vi "IMAQ-MWT (HOST).vi"() -> ()   [LabVIEW 2020]
uses:
  Modules/Common/Controls (HOST)/Image Size.ctl
  Modules/Common/Controls (HOST)/REF.ctl
  Modules/Common/Controls (HOST)/Image Queue Bundle.ctl
  Modules/Common/Controls (HOST)/Data to Disk Bundle.ctl
  Modules/Common/Controls (HOST)/File Name Prefix.ctl
  Modules/Common/Controls (HOST)/FPGA REF (MWT).ctl
  Modules/Common/Controls (HOST)/Experiment Mode.ctl
  Modules/Common/Controls (HOST)/Main States.ctl
  Modules/Common/Controls (HOST)/GUI Param.ctl
  Modules/Common/Controls (HOST)/Capture Background Image.ctl
  Modules/Common/Controls (HOST)/IMAQ Parameters.ctl
  Modules/Common/Controls (HOST)/File REF.ctl
  <vilib>/vision/Avi.llb/IMAQ AVI2 Refnum.ctl
  Modules/Common/Controls (HOST)/Load Parameters.ctl
  <vilib>/DAQmx/write.llb/DAQmx Write (Analog 2D DBL NChan NSamp).vi
  <vilib>/Utility/error.llb/Error Cluster From Error Code.vi
  <vilib>/rvi/errors/niLvFpgaAdjustHostInterfaceError.vi
  <vilib>/FPGAPlugInAG/Dynamic/niLvFpga_Close_Dynamic.vi
  <vilib>/Utility/file.llb/Read Delimited Spreadsheet (string).vi
  <vilib>/DAQmx/miscellaneous.llb/DAQmx Fill In Error Info.vi
  <vilib>/rvi/interface/nirviReadWriteControl/nirviReadWriteControl.xnode
  <vilib>/rvi/interface/nirviCloseFPGA/nirviCloseFPGA.xnode
  NiFpgaLv.dll
  <vilib>/rvi/interface/Simulation/niFpgaSimulationCallBeginRW.vi
  <vilib>/httpClient/LabVIEWHTTPClient.lvlib
panel:
  in  "Array Type":dbl[](array[numeric])
  in  "Record video?":bool=TRUE
  in  "File Path":path=path "D:/MWT/Data"
  in  "Display Type":enum16{"Live", "Background", "Background-Live"}(ring)
  in  "Display Frame Rate (Hz)":u32=5
  out "flipFlag":refnum<queue>
  out "Files Loaded":bool
  out "vReset":refnum<queue>
  out "FNP":T1={"DateTimeStamp"="DateTimeStamp", "Genotype 1"="genotype1", "Genotype 2"="genotype2", "Rig Name"="t21", "STIM Mode"="stimulationMode", "Light Intensity (%)"=100, "Pixel Resolution (um/pixel)"=100.0, "Gamma"=0.2, "Yoked File Name"="none", "Yoked File Enable"=FALSE, "Output Folder Name"=path "", "Frame Number"=0, "Time Stamp (us)"=0, "Exp STOP"=0, "Contour"=[], "SPINE"=[], "Larvae ID"=[], "Larvae Valid?"=[], "Image Height"=0, "Image Width"=0, "Pixel Intensity Low"=0, "Pixel Intensity High"=0, "Box Side Low"=0, "Box Side High"=0, "Box W+L Low"=0, "Box W+L High"=0, "Area Low"=0, "Area High"=0, "N SPINE"=0, "BG SUB TH"=0, "Min Contour Points"=0, "STIM Array"=[], "Stimulus Label Array"=[], "Flip Laravae ID"=[], "IR Intensity"=0}
  out "Load Options":bool
  in  "Load Settings":bool
  out "DLL Input Param":T1={"DateTimeStamp"="DateTimeStamp", "Genotype 1"="genotype1", "Genotype 2"="genotype2", "Rig Name"="t21", "STIM Mode"="stimulationMode", "Light Intensity (%)"=100, "Pixel Resolution (um/pixel)"=100.0, "Gamma"=0.2, "Yoked File Name"="none", "Yoked File Enable"=FALSE, "Output Folder Name"=path "", "Frame Number"=0, "Time Stamp (us)"=0, "Exp STOP"=0, "Contour"=[], "SPINE"=[], "Larvae ID"=[], "Larvae Valid?"=[], "Image Height"=0, "Image Width"=0, "Pixel Intensity Low"=0, "Pixel Intensity High"=0, "Box Side Low"=0, "Box Side High"=0, "Box W+L Low"=0, "Box W+L High"=0, "Area Low"=0, "Area High"=0, "N SPINE"=0, "BG SUB TH"=0, "Min Contour Points"=0, "STIM Array"=[], "Stimulus Label Array"=[], "Flip Laravae ID"=[], "IR Intensity"=0}
  in  "Tab Control":T2(tab)
  in  "Image Size":T3={"Height"=3072, "Width"=3200}
  in  "Experiment Mode":T4
  in  "Pixel Intensity Range":cluster{"Low":u8, "High":u8}={"Low"=25, "High"=135}
  in  "Exp. Time (S)":dbl=120.0
  out "Frame Rate":u32
  out "Frame #":u32
  in  "Stop Button":bool
  in  "Go":bool
  in  "Box Side (Pixels)":cluster{"Low":u32, "High":u32}={"Low"=6, "High"=200}
  out "# Objects":i32
  in  "Subtract BG":bool=TRUE
  in  "Capture BG":bool
  in  "Box W + L (Pixels)":cluster{"Low":u32, "High":u32}={"Low"=12, "High"=200}
  in  "Area (Pixels)":cluster{"Low":u32, "High":u32}={"Low"=500, "High"=3500}
  in  "Replay Interval (ms)":u32=1000
  in  "BG Type":bool=TRUE
  in  "Movie File Path":path=path "E:/Rawdata/72F11-Gal4xUAS-CsChrimson_20180513_192634.dbde"
  in  "Swap Bytes":bool
  in  "Load Stimulus":bool
  in  "STIM 10":dbl caption="unused"
  in  "STIM 9":dbl caption="unused"
  in  "STIM 8":dbl caption="unused"
  in  "STIM 7":dbl caption="unused"
  in  "STIM 6":dbl caption="unused"
  in  "STIM 5":dbl caption="unused"
  in  "STIM 4":dbl caption="testing_stim_ISI"
  in  "STIM 3":dbl caption="testing_stim_duration"
  in  "STIM 2":dbl caption="nOf_testing_stims"
  in  "STIM 1":dbl caption="Waiting_Time"
  in  "Yoke File Name":path=path "none"
  in  "Light Intensity (%)":i32=100
  in  "Yoked File Enable":bool
  in  "Save Stimulus":bool
  in  "Genotype 2":u16(ring) items=["empty-GAL4(attp2)", "UAS-CsChrimson", "LexAop-dTrpA1 VK5", " QUAS-CsCrimson(attp18)", " QUAS-dTrpA1(VK5)", " LexAop-CsChrimson (attp18)", " LexAop-CsChrimson VK5", " UAS-dTrpA1", "UAS-CsChrimsonTsh-Gal80", "UAS-CsChrimsonTH-Gal80", "UAS-CsChrimsonDdc-Gal4"]
  in  "STIM Mode":u16(ring) items=["open_loop_red", "always_on", "left_bend_continuous", "right_bend_continuous", "always_off", "random_bend_continuous_left", "random_bend_continuous_right", "bend_continuous", "forward_crawl_continuous", "open_loop_ir", "open_loop_ir_roll_dmd", "automated_assoc_learn", "two_alternatives_bend_continuous", "pulsed_ir", "DMD_IR_learning", "just_pulsed_DMD", "DMD_light_steps"]
  in  "Genotype 1":u16(ring) items=["72F11-Gal4", "72F11-LexA JK22C", " 72F11-QF2(attp2)", "11F02-Gal4", " 13xLexAop-CsChrimson_Or42b-LexA(JK22C)", " 13xLexAop-CsChrimson(attp18)_Or42b-LexA(JK22C)(ATR-)", " 13xLexAop-CsChrimson(attp18)_Or42b-LexA(JK22C)", " Or42b-LexA(JK22C)", " Or42b-Gal4", "SS04261", "58E02-Gal4", "ppk19-Gal4", "Ddc-Gal4-HL8-3D", "attP2", "w1118", "Tph-Gal4", "69F06-Gal4", "eg_gal4", "TH-Gal4", "69E06-LexALexAop-TrpA"]
  in  "Rig Name":u16(ring) items=["t21"]
  in  "Stimulus File":path=path "C:/MWT/Stimulation_Default.ini"
  in  "Settings File":path=path "C:/MWT/Settings_Default.ini"
  in  "Gamma":dbl=0.2 format="%#_13g"
  in  "Min Contour Points":u16=127
  in  "N Spine Points":fxp<+,8,8>=41.0
  in  "Pixel Resolution (um/Pixel)":dbl=40.69 format="%#_13g"
  in  "BG SUB TH":i16=50
  in  "Save Settings":bool
  in  "Cycle Time (ms)":i32=50
  in  "LASER Intensity (%)":dbl=40.0 min=0.0 max=100.0 format="%.2f"
  out "Max. LASER Power (W)":dbl format="%#.2f"
  in  "Temperature Range (High)":dbl=45.0
  in  "Temperature Range (Low)":dbl=20.0
  out "Intensity Graph":dbl[][](graph)
  out "Larvae 8":u32
  out "Larvae 7":u32
  out "Larvae 6":u32
  out "Larvae 5":u32
  out "Larvae 4":u32
  out "Larvae 3":u32
  out "Larvae 2":u32
  out "Larvae 1":u32
  out "BG Image":u8[][](array[numeric])
  out "Larvae 8":cluster{"Array":i32[], "Array":i32[]}[](graph)
  out "Larvae 7":cluster{"Array":i32[], "Array":i32[]}[](graph)
  out "Larvae 6":cluster{"Array":i32[], "Array":i32[]}[](graph)
  out "Larvae 5":cluster{"Array":i32[], "Array":i32[]}[](graph)
  out "Larvae 4":cluster{"Array":i32[], "Array":i32[]}[](graph)
  out "Larvae 3":cluster{"Array":i32[], "Array":i32[]}[](graph)
  out "Larvae 2":cluster{"Array":i32[], "Array":i32[]}[](graph)
  out "Larvae 1":cluster{"Array":i32[], "Array":i32[]}[](graph)
  out "Exp. Status":string="Camera Connected"
  out "REF":T5
  out "Command Q":refnum<queue>
  out "Display":T8(plugin-control)
  out "Stopped?":bool
  # "Real Time Multi Worm Tracker"
types:
  T1 = typedef "File Name Prefix.ctl" = cluster{"DateTimeStamp":string, "Genotype 1":string, "Genotype 2":string, "Rig Name":string, "STIM Mode":string, "Light Intensity (%)":i32, "Pixel Resolution (um/pixel)":dbl, "Gamma":dbl, "Yoked File Name":string, "Yoked File Enable":bool, "Output Folder Name":path, "Frame Number":u64, "Time Stamp (us)":u64, "Exp STOP":i32, "Contour":cluster{"X":i32[], "Y":i32[]}[], "SPINE":cluster{"X":dbl[], "Y":dbl[]}[], "Larvae ID":u32[], "Larvae Valid?":bool[], "Image Height":i32, "Image Width":i32, "Pixel Intensity Low":i32, "Pixel Intensity High":i32, "Box Side Low":i32, "Box Side High":i32, "Box W+L Low":i32, "Box W+L High":i32, "Area Low":i32, "Area High":i32, "N SPINE":i32, "BG SUB TH":i32, "Min Contour Points":i32, "STIM Array":dbl[], "Stimulus Label Array":u8[], "Flip Laravae ID":i32[], "IR Intensity":i32}
  T2 = enum32{"Experiment Setup", "Options", "Settings", "Heat Cam"}
  T3 = typedef "Image Size.ctl" = cluster{"Height":u16, "Width":u16}
  T4 = typedef "Experiment Mode.ctl" = enum16{"Live", "Replay"}
  T5 = typedef "REF.ctl" = cluster{"Queue REF":T6, "FPGA REF (MWT)":T7}
  T6 = typedef "Image Queue Bundle.ctl" = cluster{"Disk Image":refnum<queue>, "Image Blocks":refnum<queue>, "Display Image":refnum<queue>, "BG Image":refnum<queue>, "Tag Image":refnum<queue>, "DLL Input":refnum<queue>, "DMD Input":refnum<queue>, "GALVO Input":refnum<queue>, "Save Image":refnum<queue>}
  T7 = typedef "FPGA REF (MWT).ctl" = refnum<k20>
  T8 = typedef "IMAQ Image.ctl" = refnum<image>
  T9 = enum8{"Enabled", "Disabled", "Disabled and Grayed Out"}
  T10 = typedef "Main States.ctl" = enum16{"Open FPGA", "Initialize", "Preview", "Acquire Images", "STOP"}
  T11 = typedef "GUI Param.ctl" = cluster{"Image Width":u16, "Image Height":u16, "Pixel Intensity Low":u8, "Pixel Intensity High":u8, "Box Side Low":u32, "Box Side High":u32, "Box W+L Low":u32, "Box W+L High":u32, "Area Low":u32, "Area High":u32, "BG SUB TH":i16, "N Spine Points":fxp<+,8,8>, "Min Contour Points":u16, "Pixel Resolution (um/Pixel)":dbl, "Gamma":dbl}
  T12 = typedef "Load Parameters.ctl" = enum16{"Load Options", "Load Settings", "Load Stimulus", "STIM MODE"}
  T13 = typedef "IMAQ Parameters.ctl" = cluster{"File REF":T14, "Frame Data":cluster{"Width":u32, "Height":u32, "Frames Per Second":u32, "Codec":string}, "File Type":string, "Experiment Mode":T4, "Movie File Path":path}
  T14 = typedef "File REF.ctl" = cluster{"AVI REF":T15, "DBDE REF":refnum<file>}
  T15 = typedef "IMAQ AVI2 Refnum.ctl" = refnum<k20>
  T16 = typedef "Data to Disk Bundle.ctl" = cluster{"Frame Number":u64, "Time Stamp (us)":u64, "Image Data":u64[], "Contour":u32[], "Raw Image REF":refnum<data-value>, "Block Image REF":refnum<data-value>, "Block Box":u64[], "SPINE":u32[], "HT Angle":u64[], "Block Position":u64[], "SPINE Count":u32[], "Contour Count":u32[], "SPINE DIR":u8[]}
  T17 = enum16{"open", "replace", "create", "open or create", "replace or create", "replace or create with confirmation"}
  T18 = enum16{"fire", "rainbow", "gray", "inverse gray", "ice", "original"}
  T19 = typedef "Capture Background Image.ctl" = enum16{"Wait for UI", "Acquire Image", "Save Image", "Download Image"}
  T20 = enum16{"big-endian, network order", "native, host order", "little-endian"}
  T21 = typedef "IR GALVO Cal Data.ctl" = cluster{"G1X":dbl[][], "G1Y":dbl[][], "G2X":dbl[][], "G2Y":dbl[][], "G3X":dbl[][], "G3Y":dbl[][], "G4X":dbl[][], "G4Y":dbl[][], "G1 Intensity":dbl[][], "G2 Intensity":dbl[][], "G3 Intensity":dbl[][], "G4 Intensity":dbl[][], "L1 POWER":dbl[]}
  T22 = typedef "DMD Intensity Cal Param.ctl" = cluster{"X2":dbl, "X1":dbl, "C":dbl}
  T23 = typedef "imagedata.ctl" = cluster{"image type":i32, "image depth":i32, "image":u8[], "mask":u8[], "colors":u32[], "Rectangle":cluster{"left":i16, "top":i16, "right":i16, "bottom":i16}}
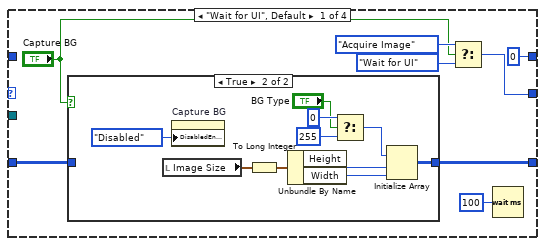
[diagram p17: hidden frame]
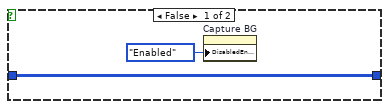
[diagram p18: hidden frame]
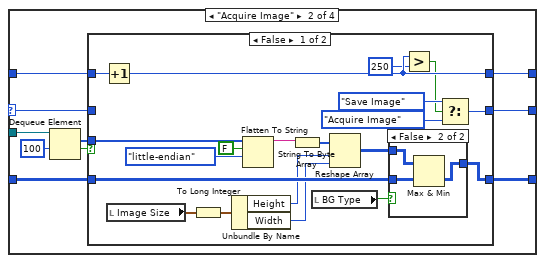
[diagram p19: hidden frame]
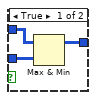
[diagram p20: hidden frame]
diagram:
  n1 = while {
    stop <- w32 stop-if-true
    # "Event Handler"
    n2 = event shown="[1] \"Go\": Value Change" {
      selector: _ -> [_ _ _ _ _ _ _ _ _ _ _]
      dyn-events: _ -> [_ _ _ _ _ _ _ _ _ _ _]
      timeout: 100 -> [_ _ _ _ _ _ _ _ _ _ _]
      event Timeout {
        n3 = event-data() -> ()  [unwired: 1 in, 1 out]
      }
      event "Go": Value Change {
        n4 = event-data() -> ("NewVal"=w33:bool)  [unwired: 1 in, 5 out]
        n5 = case shown="True" w33 {
          frame False {
          }
          frame True {
            n6 = property on="Go" class="Bool (strict)"("DisabledEnum"=T9."Disabled" ("Disabled")) -> ()  [unwired: 2 in, 2 out]
          }
        }
      }
      event "Stop Button": Value Change {
        n7 = event-data() -> ("NewVal"=w35:bool)  [unwired: 1 in]
        n8 = case shown="True" w35 {
          frame False {
          }
          frame True {
            n9 = local read "Command Q"() -> (w37:refnum<queue>)
            n10 = Enqueue Element(queue=w37, element="") -> ()  [unwired: 2 in, 3 out]
          }
        }
      }
      event "Load Options": Value Change {
        n11 = event-data() -> ()  [unwired: 1 in, 1 out]
        n12 = call "Read Options Selection (SubVI).vi"() -> ("Options Selection"=w39:i32[])  [unwired: 11 in]
        n13 = call-poly <vilib>:"Read Delimited Spreadsheet.vi"("file path (dialog if empty)"=path "C:/MWT/Options.csv", "delimiter (\\t)"="," ("delimiter (\\t)")) -> ("all rows"=w54:string[][])  [unwired: 8 in, 5 out]
        n14 = Index Array(array=w54, index (row) #1=0 ("index (row)"), index (row) #2=1 ("index (row)"), index (row) #3=2 ("index (row)"), index (row) #4=3 ("index (row)")) -> (element #1=w45:string[], element #2=w52:string[], element #3=w51:string[], element #4=w50:string[])  [unwired: 4 in]
        n15 = call "Extract Ring Text (SubVI).vi"("Spreadsheet String"=w45) -> ("Output String"=w44:string[])  [unwired: 10 in]
        n16 = call "Extract Ring Text (SubVI).vi"("Spreadsheet String"=w52) -> ("Output String"=w43:string[])  [unwired: 10 in]
        n17 = call "Extract Ring Text (SubVI).vi"("Spreadsheet String"=w51) -> ("Output String"=w42:string[])  [unwired: 10 in]
        n18 = call "Extract Ring Text (SubVI).vi"("Spreadsheet String"=w50) -> ("Output String"=w41:string[])  [unwired: 10 in]
        n19 = property on="Rig Name" class="Ring (strict)"("Strings []"=w44) -> ()  [unwired: 2 in, 2 out]
        n20 = property on="Genotype 1" class="Ring (strict)"("Strings []"=w43) -> ()  [unwired: 2 in, 2 out]
        n21 = property on="Genotype 2" class="Ring (strict)"("Strings []"=w42) -> ()  [unwired: 2 in, 2 out]
        n22 = property on="STIM Mode" class="Ring (strict)"("Strings []"=w41) -> (error out=w40:errorcluster)  [unwired: 2 in, 1 out]
        n23 = for {
          tunnel: w40 -> [_]
          tunnel: w39 -> [w56] mode=indexing
          i -> [w57]
          n24 = case shown="2" w57 {
            tunnel: w56 -> [w59 w61 w63]
            frame 0, Default {
              n25 = To Unsigned Word Integer(number=w59) -> (unsigned 16bit integer=w58:u16)
              n26 = local write "Genotype 1"(w58) -> ()
            }
            frame 1 {
              n27 = To Unsigned Word Integer(number=w61) -> (unsigned 16bit integer=w60:u16)
              n28 = local write "Genotype 2"(w60) -> ()
            }
            frame 2 {
              n29 = To Unsigned Word Integer(number=w63) -> (unsigned 16bit integer=w62:u16)
              n30 = local write "STIM Mode"(w62) -> ()
            }
          }
        }
        "Load Options" <- FALSE ("Load Options")
      }
      event "Save Settings": Value Change {
        n31 = event-data() -> ("NewVal"=w64:bool)  [unwired: 1 in]
        n32 = case shown="True" w64 {
          frame False {
          }
          frame True {
            n33 = local read "Box Side (Pixels)"() -> (w77:cluster{"Low":u32, "High":u32})
            n34 = local read "Box W + L (Pixels)"() -> (w74:cluster{"Low":u32, "High":u32})
            n35 = local read "Pixel Resolution (um/Pixel)"() -> (w68:dbl)
            n36 = local read "Image Size"() -> (w85:T3)
            n37 = local read "Pixel Intensity Range"() -> (w80:cluster{"Low":u8, "High":u8})
            n38 = local read "Area (Pixels)"() -> (w71:cluster{"Low":u32, "High":u32})
            n39 = local read "N Spine Points"() -> (w69:fxp<+,8,8>)
            n40 = local read "Min Contour Points"() -> (w67:u16)
            n41 = local read "Gamma"() -> (w66:dbl)
            n42 = local read "BG SUB TH"() -> (w70:i16)
            n43 = Unbundle By Name(w85) -> ("Width"=w84:u16, "Height"=w83:u16)
            n44 = Unbundle By Name(w80) -> ("Low"=w82:u8, "High"=w81:u8)
            n45 = Unbundle By Name(w77) -> ("Low"=w79:u32, "High"=w78:u32)
            n46 = Unbundle By Name(w74) -> ("Low"=w76:u32, "High"=w75:u32)
            n47 = Unbundle By Name(w71) -> ("Low"=w73:u32, "High"=w72:u32)
            n48 = Bundle By Name(cluster=T11 {"Image Width"=3072, "Image Height"=3072, "Pixel Intensity Low"=25, "Pixel Intensity High"=135, "Box Side Low"=6, "Box Side High"=200, "Box W+L Low"=12, "Box W+L High"=200, "Area Low"=500, "Area High"=3500, "BG SUB TH"=10, "N Spine Points"=11.0, "Min Contour Points"=127, "Pixel Resolution (um/Pixel)"=40.69, "Gamma"=0.2} ("GUI Parameters"), "Image Width"=w84, "Image Height"=w83, "Pixel Intensity Low"=w82, "Pixel Intensity High"=w81, "Box Side Low"=w79, "Box Side High"=w78, "Box W+L Low"=w76, "Box W+L High"=w75, "Area Low"=w73, "Area High"=w72, "BG SUB TH"=w70, "N Spine Points"=w69, "Min Contour Points"=w67, "Pixel Resolution (um/Pixel)"=w68, "Gamma"=w66) -> (w86:T11)
            n49 = local read "Settings File"() -> (w65:path)
            n50 = call "Save GUI Settings (SubVI).vi"("Settings File Name"=w65, "GUI Parameters"=w86) -> ()  [unwired: 10 in]
            n51 = call "Save Settings File Name (SubVI).vi"("Settings File Name"=w65) -> ()  [unwired: 11 in]
          }
        }
      }
      event "Settings File", "Load Settings": Value Change {
        n52 = event-data() -> ()  [unwired: 1 in, 6 out]
        n53 = local read "Settings File"() -> (w88:path)
        n54 = call "Read GUI Settings (SubVI).vi"("File Path"=w88) -> ("GUI Parameters"=w110:T11)  [unwired: 10 in]
        n55 = Unbundle By Name(w110) -> ("BG SUB TH"=w111:i16, "N Spine Points"=w112:fxp<+,8,8>, "Min Contour Points"=w113:u16, "Pixel Resolution (um/Pixel)"=w114:dbl, "Gamma"=w115:dbl)
        n56 = Unbundle By Name(w110) -> ("Image Width"=w92:u16, "Image Height"=w93:u16)
        n57 = Unbundle By Name(w110) -> ("Pixel Intensity Low"=w95:u8, "Pixel Intensity High"=w94:u8)
        n58 = Unbundle By Name(w110) -> ("Box Side Low"=w99:u32, "Box Side High"=w98:u32)
        n59 = Unbundle By Name(w110) -> ("Box W+L Low"=w103:u32, "Box W+L High"=w102:u32)
        n60 = Unbundle By Name(w110) -> ("Area Low"=w106:u32, "Area High"=w107:u32)
        n61 = Bundle By Name(cluster=T3 {"Height"=3072, "Width"=3072} ("Image Size"), "Width"=w92, "Height"=w93) -> (w91:T3)
        n62 = Bundle By Name(cluster=cluster{"Low":u8, "High":u8} {"Low"=25, "High"=135} ("Pixel Intensity Range"), "Low"=w95, "High"=w94) -> (w96:cluster{"Low":u8, "High":u8})
        n63 = Bundle By Name(cluster=cluster{"Low":u32, "High":u32} {"Low"=6, "High"=200} ("Box Side (Pixels)"), "Low"=w99, "High"=w98) -> (w100:cluster{"Low":u32, "High":u32})
        n64 = Bundle By Name(cluster=cluster{"Low":u32, "High":u32} {"Low"=12, "High"=200} ("Box W + L (Pixels)"), "Low"=w103, "High"=w102) -> (w105:cluster{"Low":u32, "High":u32})
        n65 = Bundle By Name(cluster=cluster{"Low":u32, "High":u32} {"Low"=500, "High"=3500} ("Area (Pixels)"), "Low"=w106, "High"=w107) -> (w109:cluster{"Low":u32, "High":u32})
        n66 = local write "Pixel Resolution (um/Pixel)"(w114) -> ()
        n67 = local write "N Spine Points"(w112) -> ()
        n68 = local write "Min Contour Points"(w113) -> ()
        n69 = local write "Gamma"(w115) -> ()
        n70 = local write "BG SUB TH"(w111) -> ()
        n71 = local write "Box Side (Pixels)"(w100) -> ()
        n72 = local write "Box W + L (Pixels)"(w105) -> ()
        n73 = local write "Image Size"(w91) -> ()
        n74 = local write "Pixel Intensity Range"(w96) -> ()
        n75 = local write "Area (Pixels)"(w109) -> ()
        n76 = local write "Load Settings"(FALSE ("Load Settings")) -> ()
      }
      event "Save Stimulus": Value Change {
        n77 = event-data() -> ("NewVal"=w116:bool)  [unwired: 1 in]
        n78 = case shown="True" w116 {
          frame False {
          }
          frame True {
            n79 = Build Array("STIM 1", "STIM 2", "STIM 3", "STIM 4", "STIM 5", "STIM 6", "STIM 7", "STIM 8", "STIM 9", "STIM 10") -> (w118:dbl[])
            n80 = property on="STIM Mode" class="Ring (strict)"() -> ("RingText.Text"=w117:string)  [unwired: 2 in, 2 out]
            n81 = local read "Stimulus File"() -> (w119:path)
            n82 = call "Save Stimulus File Name (SubVI).vi"("Stimulus File Name"=w119) -> ()  [unwired: 11 in]
            n83 = call "Save Stimulus Parameters (SubVI).vi"("STIM MODE"=w117, "Stimulus File Name"=w119, "STIM Parameters"=w118) -> ()  [unwired: 9 in]
          }
        }
      }
      event "Load Stimulus": Value Change {
        n84 = event-data() -> ("NewVal"=w130:bool)  [unwired: 1 in]
        n85 = case shown="True" w130 {
          frame False {
          }
          frame True {
            n86 = flat-sequence {
              tunnel: [w137] -> w132
              tunnel: [w133] -> w131
              tunnel: w132 -> [w165]
              tunnel: w131 -> [w163]
              frame #0 {
                n87 = local read "Stimulus File"() -> (w140:path)
                n88 = local write "Load Stimulus"(FALSE ("Load Stimulus")) -> ()
                n89 = property on="STIM Mode" class="Ring (strict)"() -> ("Strings []"=w134:string[])  [unwired: 2 in, 2 out]
                n90 = call "Load Stimulus Parameters (SubVI).vi"("Stimulus File Name"=w140) -> ("STIM MODE"=w133:string, "STIM Param"=w137:dbl[])  [unwired: 9 in]
                n91 = Search 1D Array(1D array=w134, element=w133) -> (index of element=w136:i32)  [unwired: 1 in]
                n92 = call "Read Stim Mode Labels (SubVI).vi"("STIM MODE"=w133) -> ("Label"=w138:string[])  [unwired: 10 in]
                n93 = Index Array(array=w137) -> (element #1=w150:dbl, element #2=w149:dbl, element #3=w148:dbl, element #4=w147:dbl, element #5=w146:dbl, element #6=w145:dbl, element #7=w144:dbl, element #8=w143:dbl, element #9=w142:dbl, element #10=w141:dbl)  [unwired: 10 in]
                n94 = To Unsigned Word Integer(number=w136) -> (unsigned 16bit integer=w135:u16)
                n95 = for {
                  tunnel: w138 -> [w151] mode=indexing
                  i -> [w152]
                  n96 = case shown="10" w152 {
                    tunnel: w151 -> [_ w153 w154 w155 w156 w157 w158 w159 w160 w161 w162]
                    frame 0, Default {
                    }
                    frame 1 {
                      n97 = property on="STIM 1" class="DigNum (strict)"("Caption.Text"=w153) -> ()  [unwired: 2 in, 2 out]
                    }
                    frame 2 {
                      n98 = property on="STIM 2" class="DigNum (strict)"("Caption.Text"=w154) -> ()  [unwired: 2 in, 2 out]
                    }
                    frame 3 {
                      n99 = property on="STIM 3" class="DigNum (strict)"("Caption.Text"=w155) -> ()  [unwired: 2 in, 2 out]
                    }
                    frame 4 {
                      n100 = property on="STIM 4" class="DigNum (strict)"("Caption.Text"=w156) -> ()  [unwired: 2 in, 2 out]
                    }
                    frame 5 {
                      n101 = property on="STIM 5" class="DigNum (strict)"("Caption.Text"=w157) -> ()  [unwired: 2 in, 2 out]
                    }
                    frame 6 {
                      n102 = property on="STIM 6" class="DigNum (strict)"("Caption.Text"=w158) -> ()  [unwired: 2 in, 2 out]
                    }
                    frame 7 {
                      n103 = property on="STIM 7" class="DigNum (strict)"("Caption.Text"=w159) -> ()  [unwired: 2 in, 2 out]
                    }
                    frame 8 {
                      n104 = property on="STIM 8" class="DigNum (strict)"("Caption.Text"=w160) -> ()  [unwired: 2 in, 2 out]
                    }
                    frame 9 {
                      n105 = property on="STIM 9" class="DigNum (strict)"("Caption.Text"=w161) -> ()  [unwired: 2 in, 2 out]
                    }
                    frame 10 {
                      n106 = property on="STIM 10" class="DigNum (strict)"("Caption.Text"=w162) -> ()  [unwired: 2 in, 2 out]
                    }
                  }
                }
                n107 = local write "STIM Mode"(w135) -> ()
                n108 = local write "STIM 1"(w150) -> ()
                n109 = local write "STIM 2"(w149) -> ()
                n110 = local write "STIM 3"(w148) -> ()
                n111 = local write "STIM 4"(w147) -> ()
                n112 = local write "STIM 5"(w146) -> ()
                n113 = local write "STIM 6"(w145) -> ()
                n114 = local write "STIM 7"(w144) -> ()
                n115 = local write "STIM 8"(w143) -> ()
                n116 = local write "STIM 9"(w142) -> ()
                n117 = local write "STIM 10"(w141) -> ()
              }
              frame #1 {
                n118 = for {
                  N: 10 -> [_]
                  tunnel: [w169] -> w164 mode=concatenating
                  i -> [w173]
                  n119 = case shown="0, Default" w173 {
                    tunnel: [w174 w175 w176 w177 w178 w179 w180 w181 w182 w183] -> w172
                    frame 0, Default {
                      n120 = property on="STIM 1" class="DigNum (strict)"() -> ("Caption.Text"=w174:string)  [unwired: 2 in, 2 out]
                    }
                    frame 1 {
                      n121 = property on="STIM 2" class="DigNum (strict)"() -> ("Caption.Text"=w175:string)  [unwired: 2 in, 2 out]
                    }
                    frame 2 {
                      n122 = property on="STIM 3" class="DigNum (strict)"() -> ("Caption.Text"=w176:string)  [unwired: 2 in, 2 out]
                    }
                    frame 3 {
                      n123 = property on="STIM 4" class="DigNum (strict)"() -> ("Caption.Text"=w177:string)  [unwired: 2 in, 2 out]
                    }
                    frame 4 {
                      n124 = property on="STIM 5" class="DigNum (strict)"() -> ("Caption.Text"=w178:string)  [unwired: 2 in, 2 out]
                    }
                    frame 5 {
                      n125 = property on="STIM 6" class="DigNum (strict)"() -> ("Caption.Text"=w179:string)  [unwired: 2 in, 2 out]
                    }
                    frame 6 {
                      n126 = property on="STIM 7" class="DigNum (strict)"() -> ("Caption.Text"=w180:string)  [unwired: 2 in, 2 out]
                    }
                    frame 7 {
                      n127 = property on="STIM 8" class="DigNum (strict)"() -> ("Caption.Text"=w181:string)  [unwired: 2 in, 2 out]
                    }
                    frame 8 {
                      n128 = property on="STIM 9" class="DigNum (strict)"() -> ("Caption.Text"=w182:string)  [unwired: 2 in, 2 out]
                    }
                    frame 9 {
                      n129 = property on="STIM 10" class="DigNum (strict)"() -> ("Caption.Text"=w183:string)  [unwired: 2 in, 2 out]
                    }
                  }
                  n130 = Concatenate Strings(w172, "," ("string")) -> (w171:string)
                  n131 = String To Byte Array(string=w171) -> (unsigned byte array=w169:u8[])
                }
                n132 = local read "FNP"() -> (w167:T1)
                n133 = Bundle By Name(cluster=w167, "Stimulus Label Array"=w164, "STIM Array"=w165, "STIM Mode"=w163) -> (w166:T1)
                n134 = local write "FNP"(w166) -> ()
              }
            }
          }
        }
      }
      event "Display Frame Rate (Hz)": Value Change {
        n135 = event-data() -> ()  [unwired: 1 in, 6 out]
        n136 = local read "Display Frame Rate (Hz)"() -> (w184:u32)
        n137 = call "Write Contour Display Rate (SubVI).vi"("Rate (Hz)"=w184) -> ()  [unwired: 11 in]
      }
      event "STIM Mode", "Genotype 1", "Genotype 2", "Rig Name": Value Change {
        n138 = event-data() -> ()  [unwired: 1 in, 1 out]
        n139 = flat-sequence {
          frame #0 {
            n140 = property on="STIM Mode" class="Ring (strict)"() -> ("RingText.Text"=w189:string)  [unwired: 2 in, 2 out]
            n141 = call "Read Stim Mode Labels (SubVI).vi"("STIM MODE"=w189) -> ("Label"=w190:string[])  [unwired: 10 in]
            n142 = for {
              tunnel: w190 -> [w191] mode=indexing
              i -> [w192]
              n143 = case shown="10" w192 {
                tunnel: w191 -> [_ w193 w194 w195 w196 w197 w198 w199 w200 w201 w202]
                frame 0, Default {
                }
                frame 1 {
                  n144 = property on="STIM 1" class="DigNum (strict)"("Caption.Text"=w193) -> ()  [unwired: 2 in, 2 out]
                }
                frame 2 {
                  n145 = property on="STIM 2" class="DigNum (strict)"("Caption.Text"=w194) -> ()  [unwired: 2 in, 2 out]
                }
                frame 3 {
                  n146 = property on="STIM 3" class="DigNum (strict)"("Caption.Text"=w195) -> ()  [unwired: 2 in, 2 out]
                }
                frame 4 {
                  n147 = property on="STIM 4" class="DigNum (strict)"("Caption.Text"=w196) -> ()  [unwired: 2 in, 2 out]
                }
                frame 5 {
                  n148 = property on="STIM 5" class="DigNum (strict)"("Caption.Text"=w197) -> ()  [unwired: 2 in, 2 out]
                }
                frame 6 {
                  n149 = property on="STIM 6" class="DigNum (strict)"("Caption.Text"=w198) -> ()  [unwired: 2 in, 2 out]
                }
                frame 7 {
                  n150 = property on="STIM 7" class="DigNum (strict)"("Caption.Text"=w199) -> ()  [unwired: 2 in, 2 out]
                }
                frame 8 {
                  n151 = property on="STIM 8" class="DigNum (strict)"("Caption.Text"=w200) -> ()  [unwired: 2 in, 2 out]
                }
                frame 9 {
                  n152 = property on="STIM 9" class="DigNum (strict)"("Caption.Text"=w201) -> ()  [unwired: 2 in, 2 out]
                }
                frame 10 {
                  n153 = property on="STIM 10" class="DigNum (strict)"("Caption.Text"=w202) -> ()  [unwired: 2 in, 2 out]
                }
              }
            }
          }
          frame #1 {
            n154 = property on="STIM Mode" class="Ring (strict)"() -> ("RingText.Text"=w208:string)  [unwired: 2 in, 2 out]
            n155 = property on="Genotype 1" class="Ring (strict)"() -> ("RingText.Text"=w205:string)  [unwired: 2 in, 2 out]
            n156 = property on="Genotype 2" class="Ring (strict)"() -> ("RingText.Text"=w204:string)  [unwired: 2 in, 2 out]
            n157 = property on="Rig Name" class="Ring (strict)"() -> ("RingText.Text"=w203:string)  [unwired: 2 in, 2 out]
            n158 = for {
              N: 10 -> [_]
              tunnel: [w211] -> w207 mode=concatenating
              i -> [w215]
              n159 = case shown="0, Default" w215 {
                tunnel: [w216 w217 w218 w219 w220 w221 w222 w223 w224 w225] -> w214
                frame 0, Default {
                  n160 = property on="STIM 1" class="DigNum (strict)"() -> ("Caption.Text"=w216:string)  [unwired: 2 in, 2 out]
                }
                frame 1 {
                  n161 = property on="STIM 2" class="DigNum (strict)"() -> ("Caption.Text"=w217:string)  [unwired: 2 in, 2 out]
                }
                frame 2 {
                  n162 = property on="STIM 3" class="DigNum (strict)"() -> ("Caption.Text"=w218:string)  [unwired: 2 in, 2 out]
                }
                frame 3 {
                  n163 = property on="STIM 4" class="DigNum (strict)"() -> ("Caption.Text"=w219:string)  [unwired: 2 in, 2 out]
                }
                frame 4 {
                  n164 = property on="STIM 5" class="DigNum (strict)"() -> ("Caption.Text"=w220:string)  [unwired: 2 in, 2 out]
                }
                frame 5 {
                  n165 = property on="STIM 6" class="DigNum (strict)"() -> ("Caption.Text"=w221:string)  [unwired: 2 in, 2 out]
                }
                frame 6 {
                  n166 = property on="STIM 7" class="DigNum (strict)"() -> ("Caption.Text"=w222:string)  [unwired: 2 in, 2 out]
                }
                frame 7 {
                  n167 = property on="STIM 8" class="DigNum (strict)"() -> ("Caption.Text"=w223:string)  [unwired: 2 in, 2 out]
                }
                frame 8 {
                  n168 = property on="STIM 9" class="DigNum (strict)"() -> ("Caption.Text"=w224:string)  [unwired: 2 in, 2 out]
                }
                frame 9 {
                  n169 = property on="STIM 10" class="DigNum (strict)"() -> ("Caption.Text"=w225:string)  [unwired: 2 in, 2 out]
                }
              }
              n170 = Concatenate Strings(w214, "," ("string")) -> (w213:string)
              n171 = String To Byte Array(string=w213) -> (unsigned byte array=w211:u8[])
            }
            n172 = local read "FNP"() -> (w209:T1)
            n173 = Bundle By Name(cluster=w209, "Stimulus Label Array"=w207, "STIM Mode"=w208, "Genotype 1"=w205, "Genotype 2"=w204, "Rig Name"=w203) -> (w206:T1)
            n174 = local write "FNP"(w206) -> ()
          }
        }
        n175 = Build Array("Genotype 1", "Genotype 2") -> (w186:u16[])
        n176 = To Long Integer(number=w186) -> (32bit integer=w185:i32[])
        n177 = call "Save Options Selection (SubVI).vi"("Options Selection"=w185) -> ()  [unwired: 11 in]
      }
      event "Light Intensity (%)", "Yoke File Name", "Yoked File Enable", "N Spine Points", "Min Contour Points", "Gamma", "BG SUB TH", "Pixel Resolution (um/Pixel)", "Pixel Intensity Range", "Box Side (Pixels)", "Box W + L (Pixels)", "Area (Pixels)", "STIM 1", "STIM 2", "STIM 3", "STIM 4", "STIM 5", "STIM 6", "STIM 7", "STIM 8", "STIM 9", "STIM 10": Value Change {
        n178 = event-data() -> ()  [unwired: 1 in, 6 out]
        n179 = for {
          N: 10 -> [_]
          tunnel: [w267] -> w226 mode=indexing
          i -> [w268]
          n180 = case shown="9" w268 {
            tunnel: [w269 w270 w271 w272 w273 w274 w275 w276 w277 w278] -> w267
            frame 0, Default {
              n181 = local read "STIM 1"() -> (w269:dbl)
            }
            frame 1 {
              n182 = local read "STIM 2"() -> (w270:dbl)
            }
            frame 2 {
              n183 = local read "STIM 3"() -> (w271:dbl)
            }
            frame 3 {
              n184 = local read "STIM 4"() -> (w272:dbl)
            }
            frame 4 {
              n185 = local read "STIM 5"() -> (w273:dbl)
            }
            frame 5 {
              n186 = local read "STIM 6"() -> (w274:dbl)
            }
            frame 6 {
              n187 = local read "STIM 7"() -> (w275:dbl)
            }
            frame 7 {
              n188 = local read "STIM 8"() -> (w276:dbl)
            }
            frame 8 {
              n189 = local read "STIM 9"() -> (w277:dbl)
            }
            frame 9 {
              n190 = local read "STIM 10"() -> (w278:dbl)
            }
          }
        }
        n191 = local read "Pixel Intensity Range"() -> (w237:cluster{"Low":u8, "High":u8})
        n192 = local read "Box W + L (Pixels)"() -> (w243:cluster{"Low":u32, "High":u32})
        n193 = local read "Box Side (Pixels)"() -> (w240:cluster{"Low":u32, "High":u32})
        n194 = local read "Pixel Resolution (um/Pixel)"() -> (w232:dbl)
        n195 = local read "Area (Pixels)"() -> (w246:cluster{"Low":u32, "High":u32})
        n196 = local read "Image Size"() -> (w234:T3)
        n197 = local read "Min Contour Points"() -> (w252:u16)
        n198 = local read "Light Intensity (%)"() -> (w231:i32)
        n199 = local read "Yoked File Enable"() -> (w233:bool)
        n200 = local read "Yoke File Name"() -> (w265:path)
        n201 = local read "N Spine Points"() -> (w249:fxp<+,8,8>)
        n202 = local read "BG SUB TH"() -> (w251:i16)
        n203 = local read "Gamma"() -> (w230:dbl)
        n204 = Unbundle By Name(w234) -> ("Height"=w235:u16, "Width"=w236:u16)
        n205 = Unbundle By Name(w237) -> ("Low"=w238:u8, "High"=w239:u8)
        n206 = Unbundle By Name(w240) -> ("Low"=w241:u32, "High"=w242:u32)
        n207 = Unbundle By Name(w243) -> ("Low"=w244:u32, "High"=w245:u32)
        n208 = Unbundle By Name(w246) -> ("Low"=w247:u32, "High"=w248:u32)
        n209 = To Long Integer(number=w249) -> (32bit integer=w250:i32)
        n210 = To Long Integer(number=w251) -> (32bit integer=w253:i32)
        n211 = To Long Integer(number=w252) -> (32bit integer=w254:i32)
        n212 = Path To String(path=w265) -> (string=w266:string)
        n213 = To Long Integer(number=w235) -> (32bit integer=w255:i32)
        n214 = To Long Integer(number=w236) -> (32bit integer=w256:i32)
        n215 = To Long Integer(number=w238) -> (32bit integer=w257:i32)
        n216 = To Long Integer(number=w239) -> (32bit integer=w258:i32)
        n217 = To Long Integer(number=w241) -> (32bit integer=w259:i32)
        n218 = To Long Integer(number=w242) -> (32bit integer=w260:i32)
        n219 = To Long Integer(number=w244) -> (32bit integer=w261:i32)
        n220 = To Long Integer(number=w245) -> (32bit integer=w262:i32)
        n221 = To Long Integer(number=w247) -> (32bit integer=w263:i32)
        n222 = To Long Integer(number=w248) -> (32bit integer=w264:i32)
        n223 = local read "FNP"() -> (w228:T1)
        n224 = Bundle By Name(cluster=w228, "Light Intensity (%)"=w231, "Pixel Resolution (um/pixel)"=w232, "Gamma"=w230, "Yoked File Name"=w266, "Yoked File Enable"=w233, "Image Height"=w255, "Image Width"=w256, "Pixel Intensity Low"=w257, "Pixel Intensity High"=w258, "Box Side Low"=w259, "Box Side High"=w260, "Box W+L Low"=w261, "Box W+L High"=w262, "Area Low"=w263, "Area High"=w264, "N SPINE"=w250, "BG SUB TH"=w253, "Min Contour Points"=w254, "STIM Array"=w226) -> (w229:T1)
        n225 = local write "FNP"(w229) -> ()
      }
    }
    n226 = local read "Stopped?"() -> (w32:bool)
  }
  n227 = Obtain Queue(max queue size (-1, unlimited)=10, name (unnamed)="Q", element data type="" ("name (unnamed)")) -> (queue out=→"Command Q":refnum<queue>)  [unwired: 2 in, 2 out]
  n228 = Obtain Queue(name (unnamed)="flipFlag", element data type=0) -> (queue out=→"flipFlag":refnum<queue>)  [unwired: 3 in, 2 out]
  n229 = Obtain Queue(name (unnamed)="vReset", element data type=u64 0) -> (queue out=→"vReset":refnum<queue>)  [unwired: 3 in, 2 out]
  n230 = property on="Go" class="Bool (strict)"("DisabledEnum"=T9."Enabled" ("Disabled")) -> ()  [unwired: 2 in, 2 out]
  n231 = while {
    shift-right: [w288] -> _
    shift-left: _ -> [w287]
    shift-right: [w279] -> _
    shift-left: Main_States."Open FPGA" -> [w289]
    shift-right: [w281] -> _
    shift-left: _ -> [w280]
    stop <- w285 stop-if-true
    # "Main Loop"
    n232 = case shown="\"Initialize\"" w289 {
      tunnel: [w298 w322 w343 w361 w396] -> w288
      tunnel: w287 -> [_ w323 w343 w361 w396]
      tunnel: [Main_States."Initialize" Main_States."Preview" w357 w385 Main_States."STOP"] -> w286
      tunnel: [_ _ _ _ w398] -> w285
      tunnel: [_ _ _ _ w398] -> w284
      tunnel: [w292 w327 w350 w369 w395] -> w281
      tunnel: w280 -> [_ w334 w350 w369 w395]
      frame "Open FPGA", Default {
        # "Create initial Q References"
        n233 = call "Create FPGA Reference (DBDE) (SubVI).vi"() -> ("FPGA REF (MWT)"=w300:T7)  [unwired: 11 in]
        n234 = call "Create Q Reference (SubVI).vi"() -> ("Image Queue"=w299:T6)  [unwired: 11 in]
        n235 = while {
          shift-right: [w305] -> _
          shift-left: Load_Parameters."Load Options" -> [w306]
          stop <- w304 stop-if-true
          # "Load Settings/Options/Stimulus"
          n236 = case shown="\"Load Stimulus\"" w306 {
            tunnel: [Load_Parameters."Load Settings" Load_Parameters."Load Stimulus" Load_Parameters."STIM MODE"] -> w305
            tunnel: [_ _ TRUE] -> w304
            frame "Load Options", Default {
              n237 = Wait (ms)(milliseconds to wait=u32 100) -> ()  [unwired: 1 out]
              n238 = property on="Load Options" class="Bool (strict)"("Val(Sgnl)"=TRUE ("Value (Signaling)")) -> ()  [unwired: 2 in, 2 out]
            }
            frame "Load Settings" {
              n239 = flat-sequence {
                frame #0 {
                  n240 = call "Read Settings File Name (SubVI).vi"() -> ("Settings File Name"=w312:path)  [unwired: 11 in]
                  n241 = local write "Settings File"(w312) -> ()
                }
                frame #1 {
                  n242 = property on="Load Settings" class="Bool (strict)"("Val(Sgnl)"=TRUE ("Value (Signaling)")) -> ()  [unwired: 2 in, 2 out]
                }
              }
              n243 = Wait (ms)(milliseconds to wait=u32 100) -> ()  [unwired: 1 out]
            }
            frame "Load Stimulus" {
              n244 = flat-sequence {
                frame #0 {
                  n245 = call "Read Stimulus File Name (SubVI).vi"() -> ("Stimulus File"=w317:path)  [unwired: 11 in]
                  n246 = local write "Stimulus File"(w317) -> ()
                }
                frame #1 {
                  n247 = property on="Load Stimulus" class="Bool (strict)"("Val(Sgnl)"=TRUE ("Value (Signaling)")) -> ()  [unwired: 2 in, 2 out]
                }
              }
              n248 = Wait (ms)(milliseconds to wait=u32 500) -> ()  [unwired: 1 out]
            }
          }
        }
        n249 = while {
          stop <- w303 stop-if-true
          # "Wait until DMD parameter files are loaded"
          n250 = Wait (ms)(milliseconds to wait=u32 100) -> ()  [unwired: 1 out]
          n251 = local read "Files Loaded"() -> (w303:bool)
        }
        n252 = Bundle By Name(cluster=T5 {"Queue REF"={"Disk Image"=refnum, "Image Blocks"=refnum, "Display Image"=refnum, "BG Image"=refnum, "Tag Image"=refnum, "DLL Input"=refnum, "DMD Input"=refnum, "GALVO Input"=refnum, "Save Image"=refnum}, "FPGA REF (MWT)"=refnum}, "FPGA REF (MWT)"=w300, "Queue REF"=w299) -> (w298:T5)
        "REF" <- w298
        n253 = Bundle By Name(cluster=T13 {"File REF"={"AVI REF"=refnum, "DBDE REF"=refnum}, "Frame Data"={"Width"=0, "Height"=0, "Frames Per Second"=0, "Codec"=""}, "File Type"="", "Experiment Mode"=enum."Live", "Movie File Path"=path "D:/Movies Formatted on November 5th 2015/Clip (2) Formatted.raw"} ("Movie File Property"), "Experiment Mode"="Experiment Mode", "Movie File Path"="Movie File Path") -> (w292:T13)
        n254 = local write "Exp. Status"("Please wait! Program initializing" ("Exp. Status")) -> ()
        n255 = property on="Exp. Status" class="Str"("Text.BGColor"=u32 11842560) -> ()  [unwired: 2 in, 2 out]
      }
      frame "Initialize" {
        n256 = local read "Image Size"() -> (w325:T3)
        n257 = call "Set Mode (MWT) (SubVI).vi"("Image Size In"=w325, "REF IN"=w323, "Parameters In"=w334) -> ("REF OUT"=w326:T5, "Parameters Out"=w328:T13, "Image Size Out"=w324:T3)  [unwired: 6 in]
        n258 = local write "Image Size"(w324) -> ()
        n259 = local read "Settings File"() -> (w319:path)
        n260 = call "Initialize  (MWT) (SubVI).vi"("Min Contour Points"="Min Contour Points", "N Spline Points"="N Spine Points", "REF IN"=w326, "Settings File Name"=w319, "Parameters In"=w328) -> ("REF OUT"=w322:T5, "Parameters Out"=w327:T13, "Exp. Status"=→"Exp. Status":string, "OK?"=w330:bool)  [unwired: 3 in]
        n261 = case shown="True" w330 {
          frame False {
            n262 = property on="Exp. Status" class="Str"("Text.BGColor"=u32 16729106) -> ()  [unwired: 2 in, 2 out]
          }
          frame True {
            n263 = property on="Exp. Status" class="Str"("Text.BGColor"=u32 10601373) -> ()  [unwired: 2 in, 2 out]
            n264 = local read "Command Q"() -> (w338:refnum<queue>)
            n265 = Enqueue Element(queue=w338, element="v") -> ()  [unwired: 2 in, 3 out]
          }
        }
        n266 = property on="Go" class="Bool (strict)"("DisabledEnum"=T9."Enabled" ("Disabled")) -> ()  [unwired: 2 in, 2 out]
        n267 = property on="Experiment Mode" class="Enum (strict)"("DisabledEnum"=T9."Disabled" ("Disabled")) -> ()  [unwired: 2 in, 2 out]
        n268 = local write "Go"(FALSE ("Go")) -> ()
      }
      frame "Preview" {
        # "This is where the IR camera data is gathered from the FPGA"
        n269 = local read "Experiment Mode"() -> (w341:T4)
        n270 = local read "Image Size"() -> (w347:T3)
        n271 = call "Queue Image (MMF) (SubVI).vi"("Experiment Mode"=w341, "Image Size"=w347, "Data Bundle"=w343) -> ()  [unwired: 9 in]
        n272 = Unbundle By Name(w343) -> ("FPGA REF (MWT)"=w353:T7)
        n273 = xnode "Read/Write Control"("FPGA VI Reference In"=w353, "Pixel Intensity"="Pixel Intensity Range", "Clock Cycles Limit"=u32 10000, "Swap Bytes"="Swap Bytes") -> ("Frame Interval"=w355:u32, "Frame #"=w346:u32, "DMA Timeout"=w345:bool)  [unwired: 1 in, 2 out]
        n274 = To Double Precision Float(number=w355) -> (double precision float=w354:dbl)
        n275 = local write "Frame #"(w346) -> ()
        n276 = Divide(x=110000000.0 ("y"), y=w354) -> (x/y=w351:dbl)
        n277 = To Unsigned Long Integer(number=w351) -> (unsigned 32bit integer=w349:u32)
        n278 = case shown="True" w345 {
          frame False {
          }
          frame True {
            n279 = property on="Exp. Status" class="Str"("Text.BGColor"=u32 16729106) -> ()  [unwired: 2 in, 2 out]
            n280 = local write "Exp. Status"("Reduce Frame Rate" ("Exp. Status")) -> ()
          }
        }
        n281 = local write "Frame Rate"(w349) -> ()
        n282 = Select(t=Main_States."Acquire Images", s="Go", f=Main_States."Preview") -> (s? t:f=w357:T10)
      }
      frame "Acquire Images" {
        # "Get frame index and rate"
        # "Get image data (either live or recorded)"
        # "Has total time elapsed?"
        n283 = local read "Experiment Mode"() -> (w365:T4)
        n284 = Unbundle By Name(w369) -> ("Experiment Mode"=w368:T4)
        n285 = call "Send Image to FPGA (SubVI).vi"("Data Bundle"=w361, "Parameters"=w369) -> ("TimeStamp"=w364:u64, "Frame Number"=w363:u64, "EOF"=w383:bool)  [unwired: 11 in]
        n286 = call "Queue Image (MMF) (SubVI).vi"("TimeStamp"=w364, "Frame Number"=w363, "Experiment Mode"=w365, "Image Size"="Image Size", "Data Bundle"=w361) -> ()  [unwired: 7 in]
        n287 = call "Get Elapsed Time (SubVI).vi"("Go"=TRUE, "Experiment Time (S)"="Exp. Time (S)") -> ("Done"=w374:bool, "Time Status"=w373:string)  [unwired: 8 in]
        n288 = Or(x=w374, y=w383) -> (x .or. y?=w375:bool)
        n289 = case shown="True" w383 {
          frame False {
          }
          frame True {
            n290 = One Button Dialog(message="End of Movie Reached") -> ()  [unwired: 1 in, 1 out]
          }
        }
        n291 = case shown="\"Replay\"" w368 {
          frame "Live", Default {
          }
          frame "Replay" {
            # "Limit image upload rate to 30 Hz"
            n292 = Wait (ms)(milliseconds to wait="Replay Interval (ms)") -> ()  [unwired: 1 out]
          }
        }
        n293 = local write "Exp. Status"(w373) -> ()
        n294 = local read "Pixel Intensity Range"() -> (w367:cluster{"Low":u8, "High":u8})
        n295 = Unbundle By Name(w361) -> ("FPGA REF (MWT)"=w380:T7)
        n296 = local read "Swap Bytes"() -> (w362:bool)
        n297 = xnode "Read/Write Control"("FPGA VI Reference In"=w380, "Pixel Intensity"=w367, "Significant Angle"=fxp<+,16,3> 0.0699462890625, "Swap Bytes"=w362) -> ("Frame Interval"=w382:u32, "Frame #"=→"Frame #":u32, "DMA Timeout"=w370:bool)  [unwired: 1 in, 2 out]
        n298 = case shown="True" w370 {
          frame False {
          }
          frame True {
            n299 = property on="Exp. Status" class="Str"("Text.BGColor"=u32 16729106) -> ()  [unwired: 2 in, 2 out]
            n300 = local write "Exp. Status"("Reduce Frame Rate" ("Exp. Status")) -> ()
          }
        }
        n301 = To Double Precision Float(number=w382) -> (double precision float=w381:dbl)
        n302 = Divide(x=110000000.0 ("y"), y=w381) -> (x/y=w377:dbl)
        n303 = To Unsigned Long Integer(number=w377) -> (unsigned 32bit integer=→"Frame Rate":u32)
        n304 = Select(t=Main_States."STOP", s=w375, f=Main_States."Acquire Images") -> (s? t:f=w385:T10)
      }
      frame "STOP" {
        w398 = TRUE
        n305 = Unbundle By Name(w396) -> ("FPGA REF (MWT)"=w397:T7)
        n306 = xnode "Close FPGA VI Reference"("FPGA VI Reference In"=w397) -> ("error out"=w392:errorcluster)  [unwired: 1 in]
        n307 = call <vilib>:"Clear Errors.vi"("error in (no error)"=w392) -> ()  [unwired: 5 in, 2 out]
        n308 = local write "Exp. Status"("Experiment Complete!" ("Exp. Status")) -> ()
        n309 = property on="Experiment Mode" class="Enum (strict)"("DisabledEnum"=T9."Enabled" ("Disabled")) -> ()  [unwired: 2 in, 2 out]
      }
    }
    "Stopped?" <- w284
    n310 = Select(t=Main_States."STOP", s="Stop Button", f=w286) -> (s? t:f=w279:T10)
  }
  n311 = flat-sequence {
    tunnel: [w401] -> w24
    tunnel: w24 -> [w408]
    frame #0 {
      w404 = u32 10263708 ("Plot Area:Colors:BG Color")
      # "Make sure initialization is done"
      n312 = local read "Command Q"() -> (w405:refnum<queue>)
      n313 = local write "Stopped?"(FALSE ("Stopped?")) -> ()
      n314 = local write "Files Loaded"(FALSE ("TP")) -> ()
      n315 = property on="Larvae 1" class="XYGraph (strict)"("BG Color"=w404, "FG Color"=w404, "Frame Color"=w404) -> ()  [unwired: 2 in, 2 out]
      n316 = local write "Go"(FALSE ("Go")) -> ()
      n317 = Preview Queue Element(queue=w405) -> (element=w401:string)  [unwired: 2 in, 3 out]
    }
    frame #1 {
      n318 = Equal?(x=w408, y="v") -> (x = y?=w406:bool)
      n319 = case shown="True" w406 {
        frame False {
        }
        frame True {
          w455 = 0  # Exp STOP
          # "READ EXPERIMENT DATA FROM GUI"
          n320 = for {
            N: 10 -> [_]
            tunnel: [w471] -> w415 mode=concatenating
            i -> [w475]
            n321 = case shown="0, Default" w475 {
              tunnel: [w476 w477 w478 w479 w480 w481 w482 w483 w484 w485] -> w474
              frame 0, Default {
                n322 = property on="STIM 1" class="DigNum (strict)"() -> ("Caption.Text"=w476:string)  [unwired: 2 in, 2 out]
              }
              frame 1 {
                n323 = property on="STIM 2" class="DigNum (strict)"() -> ("Caption.Text"=w477:string)  [unwired: 2 in, 2 out]
              }
              frame 2 {
                n324 = property on="STIM 3" class="DigNum (strict)"() -> ("Caption.Text"=w478:string)  [unwired: 2 in, 2 out]
              }
              frame 3 {
                n325 = property on="STIM 4" class="DigNum (strict)"() -> ("Caption.Text"=w479:string)  [unwired: 2 in, 2 out]
              }
              frame 4 {
                n326 = property on="STIM 5" class="DigNum (strict)"() -> ("Caption.Text"=w480:string)  [unwired: 2 in, 2 out]
              }
              frame 5 {
                n327 = property on="STIM 6" class="DigNum (strict)"() -> ("Caption.Text"=w481:string)  [unwired: 2 in, 2 out]
              }
              frame 6 {
                n328 = property on="STIM 7" class="DigNum (strict)"() -> ("Caption.Text"=w482:string)  [unwired: 2 in, 2 out]
              }
              frame 7 {
                n329 = property on="STIM 8" class="DigNum (strict)"() -> ("Caption.Text"=w483:string)  [unwired: 2 in, 2 out]
              }
              frame 8 {
                n330 = property on="STIM 9" class="DigNum (strict)"() -> ("Caption.Text"=w484:string)  [unwired: 2 in, 2 out]
              }
              frame 9 {
                n331 = property on="STIM 10" class="DigNum (strict)"() -> ("Caption.Text"=w485:string)  [unwired: 2 in, 2 out]
              }
            }
            n332 = Concatenate Strings(w474, "," ("string")) -> (w473:string)
            n333 = String To Byte Array(string=w473) -> (unsigned byte array=w471:u8[])
          }
          n334 = for {
            N: 10 -> [_]
            tunnel: [w486] -> w414 mode=indexing
            i -> [w487]
            n335 = case shown="9" w487 {
              tunnel: [w488 w489 w490 w491 w492 w493 w494 w495 w496 w497] -> w486
              frame 0, Default {
                n336 = local read "STIM 1"() -> (w488:dbl)
              }
              frame 1 {
                n337 = local read "STIM 2"() -> (w489:dbl)
              }
              frame 2 {
                n338 = local read "STIM 3"() -> (w490:dbl)
              }
              frame 3 {
                n339 = local read "STIM 4"() -> (w491:dbl)
              }
              frame 4 {
                n340 = local read "STIM 5"() -> (w492:dbl)
              }
              frame 5 {
                n341 = local read "STIM 6"() -> (w493:dbl)
              }
              frame 6 {
                n342 = local read "STIM 7"() -> (w494:dbl)
              }
              frame 7 {
                n343 = local read "STIM 8"() -> (w495:dbl)
              }
              frame 8 {
                n344 = local read "STIM 9"() -> (w496:dbl)
              }
              frame 9 {
                n345 = local read "STIM 10"() -> (w497:dbl)
              }
            }
          }
          n346 = local read "Movie File Path"() -> (w461:path)
          n347 = local read "Experiment Mode"() -> (w460:T4)
          n348 = local read "Pixel Intensity Range"() -> (w451:cluster{"Low":u8, "High":u8})
          n349 = local read "Box W + L (Pixels)"() -> (w445:cluster{"Low":u32, "High":u32})
          n350 = local read "Box Side (Pixels)"() -> (w448:cluster{"Low":u32, "High":u32})
          n351 = local read "Pixel Resolution (um/Pixel)"() -> (w457:dbl)
          n352 = local read "Area (Pixels)"() -> (w442:cluster{"Low":u32, "High":u32})
          n353 = local read "Image Size"() -> (w454:T3)
          n354 = local read "Min Contour Points"() -> (w436:u16)
          n355 = property on="Genotype 1" class="Ring (strict)"() -> ("RingText.Text"=w421:string)  [unwired: 2 in, 2 out]
          n356 = property on="Genotype 2" class="Ring (strict)"() -> ("RingText.Text"=w420:string)  [unwired: 2 in, 2 out]
          n357 = property on="Rig Name" class="Ring (strict)"() -> ("RingText.Text"=w419:string)  [unwired: 2 in, 2 out]
          n358 = property on="STIM Mode" class="Ring (strict)"() -> ("RingText.Text"=w418:string)  [unwired: 2 in, 2 out]
          n359 = local read "Light Intensity (%)"() -> (w458:i32)
          n360 = local read "Yoked File Enable"() -> (w456:bool)
          n361 = local read "Yoke File Name"() -> (w423:path)
          n362 = local read "N Spine Points"() -> (w439:fxp<+,8,8>)
          n363 = local read "BG SUB TH"() -> (w437:i16)
          n364 = call "Generate Date Time Stamp (SubVI).vi"("Experiment Mode"=w460, "Movie File Path"=w461) -> ("Date Time String"=w464:string)  [unwired: 9 in]
          n365 = local read "Gamma"() -> (w459:dbl)
          n366 = Unbundle By Name(w454) -> ("Height"=w453:u16, "Width"=w452:u16)
          n367 = Unbundle By Name(w451) -> ("Low"=w450:u8, "High"=w449:u8)
          n368 = Unbundle By Name(w448) -> ("Low"=w447:u32, "High"=w446:u32)
          n369 = Unbundle By Name(w445) -> ("Low"=w444:u32, "High"=w443:u32)
          n370 = Unbundle By Name(w442) -> ("Low"=w441:u32, "High"=w440:u32)
          n371 = To Long Integer(number=w439) -> (32bit integer=w438:i32)
          n372 = To Long Integer(number=w437) -> (32bit integer=w435:i32)
          n373 = To Long Integer(number=w436) -> (32bit integer=w434:i32)
          n374 = Path To String(path=w423) -> (string=w422:string)
          n375 = To Long Integer(number=w453) -> (32bit integer=w433:i32)
          n376 = To Long Integer(number=w452) -> (32bit integer=w432:i32)
          n377 = To Long Integer(number=w450) -> (32bit integer=w431:i32)
          n378 = To Long Integer(number=w449) -> (32bit integer=w430:i32)
          n379 = To Long Integer(number=w447) -> (32bit integer=w429:i32)
          n380 = To Long Integer(number=w446) -> (32bit integer=w428:i32)
          n381 = To Long Integer(number=w444) -> (32bit integer=w427:i32)
          n382 = To Long Integer(number=w443) -> (32bit integer=w426:i32)
          n383 = To Long Integer(number=w441) -> (32bit integer=w425:i32)
          n384 = To Long Integer(number=w440) -> (32bit integer=w424:i32)
          n385 = Bundle By Name(cluster=T1 {"DateTimeStamp"="DateTimeStamp", "Genotype 1"="genotype1", "Genotype 2"="genotype2", "Rig Name"="stimulationMode", "STIM Mode"="t21", "Light Intensity (%)"=100, "Pixel Resolution (um/pixel)"=100.0, "Gamma"=0.2, "Yoked File Name"="none", "Yoked File Enable"=FALSE, "Output Folder Name"=path "", "Frame Number"=0, "Time Stamp (us)"=0, "Exp STOP"=0, "Contour"=[], "SPINE"=[], "Larvae ID"=[], "Larvae Valid?"=[], "Image Height"=0, "Image Width"=0, "Pixel Intensity Low"=0, "Pixel Intensity High"=0, "Box Side Low"=0, "Box Side High"=0, "Box W+L Low"=0, "Box W+L High"=0, "Area Low"=0, "Area High"=0, "N SPINE"=0, "BG SUB TH"=0, "Min Contour Points"=0, "STIM Array"=[], "Stimulus Label Array"=[], "Flip Laravae ID"=[], "IR Intensity"=0}, "DateTimeStamp"=w464, "Genotype 1"=w421, "Genotype 2"=w420, "Rig Name"=w419, "STIM Mode"=w418, "Light Intensity (%)"=w458, "Pixel Resolution (um/pixel)"=w457, "Gamma"=w459, "Yoked File Name"=w422, "Yoked File Enable"=w456, "Exp STOP"=w455, "Image Height"=w433, "Image Width"=w432, "Pixel Intensity Low"=w431, "Pixel Intensity High"=w430, "Box Side Low"=w429, "Box Side High"=w428, "Box W+L Low"=w427, "Box W+L High"=w426, "Area Low"=w425, "Area High"=w424, "N SPINE"=w438, "BG SUB TH"=w435, "Min Contour Points"=w434, "STIM Array"=w414, "Stimulus Label Array"=w415) -> (→"FNP":T1)
          n386 = local read "REF"() -> (w409:T5)
          n387 = Unbundle By Name(w409) -> ("Queue REF.GALVO Input"=w411:refnum<queue>)
          n388 = Unbundle By Name(w409) -> ("Queue REF.Display Image"=w468:refnum<queue>)
          n389 = Unbundle By Name(w409) -> ("Queue REF.Tag Image"=w466:refnum<queue>)
          n390 = Unbundle By Name(w409) -> ("Queue REF.BG Image"=w467:refnum<queue>)
          n391 = Unbundle By Name(w409) -> ("Queue REF.Disk Image"=w469:refnum<queue>)
          n392 = Unbundle By Name(w409) -> ("Queue REF.DLL Input"=w413:refnum<queue>)
          n393 = Unbundle By Name(w409) -> ("Queue REF.DMD Input"=w412:refnum<queue>)
          n394 = Unbundle By Name(w409) -> ("Queue REF.Save Image"=w410:refnum<queue>)
          n395 = while {
            tunnel: [w511] -> w470
            tunnel: w469 -> [w503]
            tunnel: w468 -> [w510]
            tunnel: w467 -> [w508]
            tunnel: w466 -> [w507]
            tunnel: w413 -> [w502]
            tunnel: w412 -> [w501]
            tunnel: w411 -> [w500]
            tunnel: w410 -> [w499]
            stop <- w504 stop-if-true
            # "Q Images"
            n396 = property on="Stopped?" class="Bool (strict)"() -> ("Value"=w504:bool)  [unwired: 2 in, 2 out]
            n397 = Dequeue Element(queue=w503, timeout in ms (-1)=100) -> (queue out=w506:refnum<queue>, element=w509:T16, timed out?=w505:bool)  [unwired: 1 in, 1 out]
            n398 = case shown="False" w505 {
              tunnel: w506 -> [w548 w584]
              tunnel: [w548 w584] -> w511
              tunnel: w510 -> [w547 _]
              tunnel: w509 -> [w538 _]
              tunnel: w508 -> [w546 _]
              tunnel: w507 -> [w543 _]
              tunnel: w502 -> [w529 _]
              tunnel: w501 -> [w527 _]
              tunnel: w500 -> [w526 _]
              tunnel: w499 -> [w521 _]
              tunnel: "Record video?" -> [w514 _]
              frame False {
                # "Use raw image data to output contours and spines"
                # "Queue display and tag images"
                n399 = Unbundle By Name(w538) -> ("Raw Image REF"=w545:refnum<data-value>)
                n400 = Unbundle By Name(w538) -> ("Frame Number"=w518:u64, "Time Stamp (us)"=w517:u64)
                n401 = local read "LASER Intensity (%)"() -> (w525:dbl)
                n402 = for {
                  N: 128 -> [_]
                  tunnel: [w553] -> w530 mode=indexing if=w551
                  stop <- w552 stop-if-true
                  n403 = local read "flipFlag"() -> (w555:refnum<queue>)
                  n404 = Dequeue Element(queue=w555, timeout in ms (-1)=0) -> (element=w553:i32, timed out?=w552:bool)  [unwired: 1 in, 2 out]
                  n405 = Not(x=w552) -> (.not. x?=w551:bool)
                }
                n406 = local read "Capture BG"() -> (w544:bool)
                n407 = Delete Data Value Reference(data value reference=w545) -> (data value=w516:u64[])  [unwired: 1 in, 1 out]
                n408 = Bundle By Name(cluster=T16 {"Frame Number"=0, "Time Stamp (us)"=0, "Image Data"=[], "Contour"=[], "Raw Image REF"=refnum, "Block Image REF"=refnum, "Block Box"=[], "SPINE"=[], "HT Angle"=[], "Block Position"=[], "SPINE Count"=[], "Contour Count"=[], "SPINE DIR"=[]} ("element"), "Frame Number"=w518, "Time Stamp (us)"=w517, "Image Data"=w516) -> (w519:T16)
                n409 = local read "Go"() -> (w515:bool)
                n410 = Bundle By Name(cluster=w538, "Image Data"=w516) -> (w542:T16)
                n411 = call "Enque Image (BG) (SubVI).vi"("Enque"=w544, "Image Array"=w516, "BG Image REF"=w546) -> ()  [unwired: 9 in]
                n412 = local read "FNP"() -> (w532:T1)
                n413 = Bundle By Name(cluster=w532, "Frame Number"=w518, "Time Stamp (us)"=w517) -> (w539:T1)
                n414 = Multiply(x=w525, y=100.0) -> (x*y=w523:dbl)
                n415 = And(x=w514, y=w515) -> (x .and. y?=w513:bool)
                n416 = To Long Integer(number=w523) -> (32bit integer=w522:i32)
                n417 = case shown="True" w513 {
                  tunnel: w521 -> [_ w550]
                  tunnel: w519 -> [_ w549]
                  frame False {
                  }
                  frame True {
                    n418 = Enqueue Element(queue=w550, element=w549) -> ()  [unwired: 2 in, 3 out]
                  }
                }
                n419 = call "Enque Image (Display) (SubVI).vi"("Data Bundle"=w542, "Display Image REF"=w547) -> ()  [unwired: 10 in]
                n420 = call "Enque Image (Tag) (SubVI).vi"("Data Bundle"=w542, "Tag Image REF"=w543) -> ()  [unwired: 10 in]
                n421 = call "Construct Contour SPINE Array (SubVI).vi"("DATA Cluster"=w542) -> ("Larvae Valid?"=w533:bool[], "Larvae ID"=w534:u32[], "SPINE"=w535:cluster{"Array":dbl[], "Array":dbl[]}[], "Contour"=w536:cluster{"Array":i32[], "Array":i32[]}[], "Frame Valid?"=w528:bool)  [unwired: 6 in]
                n422 = Bundle By Name(cluster=w539, "Contour"=w536, "SPINE"=w535, "Larvae ID"=w534, "Larvae Valid?"=w533, "Flip Laravae ID"=w530, "IR Intensity"=w522) -> (w537:T1)
                n423 = local read "Go"() -> (w540:bool)
                n424 = And(x=w540, y=w528) -> (x .and. y?=w541:bool)
                n425 = case shown="True" w541 {
                  tunnel: w537 -> [_ w567]
                  tunnel: w529 -> [_ w564]
                  tunnel: w527 -> [_ w560]
                  tunnel: w526 -> [_ w558]
                  frame False {
                  }
                  frame True {
                    # "Update Queue REF.GALVO Input with current irData (from .dll)"
                    # "Update Queue REF.DMD Input with current dmdData (from .dll)"
                    # "Update Queue REF.DLL Input with current DLL Input Param"
                    n426 = feedback #1(TRUE ("Stopped?")) -> (w569:bool)
                    n427 = feedback-in #1(FALSE ("Stopped?")) -> ()
                    n428 = feedback #2() -> (w568:path)  [unwired: 1 in]
                    n429 = case shown="True" w569 {
                      tunnel: w567 -> [_ w582]
                      tunnel: [w580 w581] -> w566
                      tunnel: w568 -> [w580 _]
                      frame False {
                      }
                      frame True {
                        n430 = local read "Settings File"() -> (w583:path)
                        n431 = call "Create Output Folder (SubVI).vi"("Settings File Name"=w583, "DLL Input Param"=w582) -> ("Folder Name"=w581:path)  [unwired: 9 in]
                      }
                    }
                    n432 = feedback-in #2(w566) -> ()
                    n433 = Bundle By Name(cluster=w567, "Output Folder Name"=w566) -> (w563:T1)
                    "DLL Input Param" <- w563
                    n434 = Enqueue Element(queue=w564, element=w563, timeout in ms (-1)=100) -> ()  [unwired: 1 in, 3 out]
                    n435 = call "Send to Behavior Classifier (SubVI).vi"("DLL Input Param"=w563) -> ("dmdData"=w559:i32[], "voteRESET"=w565:u32[][], "irData"=w556:i32[])  [unwired: 16 in]
                    n436 = for {
                      tunnel: w565 -> [w575] mode=indexing
                      n437 = Index Array(array=w575) -> (element #1=w573:u32, element #2=w572:u32)  [unwired: 2 in]
                      n438 = Not Equal To 0?(x=w572) -> (x != 0?=w574:bool)
                      n439 = case shown="True" w574 {
                        tunnel: w573 -> [_ w578]
                        tunnel: w572 -> [_ w579]
                        frame False {
                        }
                        frame True {
                          n440 = Join Numbers(hi=w578, lo=w579) -> ((hi.lo)=w577:u64)
                          n441 = local read "vReset"() -> (w576:refnum<queue>)
                          n442 = Enqueue Element(queue=w576, element=w577) -> ()  [unwired: 2 in, 3 out]
                        }
                      }
                    }
                    n443 = Enqueue Element(queue=w560, element=w559, timeout in ms (-1)=100) -> ()  [unwired: 1 in, 3 out]
                    n444 = Enqueue Element(queue=w558, element=w556, timeout in ms (-1)=100) -> ()  [unwired: 1 in, 3 out]
                  }
                }
              }
              frame True {
              }
            }
          }
          n445 = Release Queue(queue=w470) -> (error out=w462:errorcluster)  [unwired: 2 in, 2 out]
          n446 = call <vilib>:"Clear Errors.vi"("error in (no error)"=w462) -> ()  [unwired: 5 in, 2 out]
        }
      }
    }
    frame #2 {
      n447 = local read "DLL Input Param"() -> (w587:T1)
      n448 = Bundle By Name(cluster=w587, "Exp STOP"=1) -> (w585:T1)
      n449 = local write "Stopped?"(FALSE ("Stopped?")) -> ()
      n450 = property on="Go" class="Bool (strict)"("DisabledEnum"=T9."Enabled" ("Disabled")) -> ()  [unwired: 2 in, 2 out]
      n451 = local write "Go"(FALSE ("Go")) -> ()
      n452 = call "Send to Behavior Classifier (SubVI).vi"("DLL Input Param"=w585) -> ()  [unwired: 16 in, 3 out]
    }
  }
  n453 = flat-sequence {
    tunnel: [w610] -> w17
    tunnel: [w609] -> w16
    tunnel: [w608] -> w15
    tunnel: [w595] -> w14
    tunnel: [w604] -> w13
    tunnel: [w593] -> w12
    tunnel: [w594] -> w11
    tunnel: [w603] -> w10
    tunnel: [w602] -> w9
    tunnel: [w601] -> w8
    tunnel: [w600] -> w7
    tunnel: [w599] -> w6
    tunnel: [w598] -> w5
    tunnel: [w597] -> w4
    tunnel: [w592] -> w2
    tunnel: [w591] -> w1
    tunnel: w17 -> [w664]
    tunnel: w16 -> [w663]
    tunnel: w15 -> [w662]
    tunnel: w14 -> [w661]
    tunnel: w13 -> [w660]
    tunnel: w12 -> [w658]
    tunnel: w11 -> [w659]
    tunnel: w10 -> [w657]
    tunnel: w9 -> [w656]
    tunnel: w8 -> [w651]
    tunnel: w7 -> [w650]
    tunnel: w6 -> [w645]
    tunnel: w5 -> [w644]
    tunnel: w4 -> [w643]
    tunnel: w2 -> [w641]
    tunnel: w1 -> [w634]
    frame #0 {
      # "Same as above, but for DMD 2"
      # "Initialise DMD 1 control, outputting DMD VI REF, STOP, and IMAGE REF"
      # "Wait for Qs to Initialized"
      n454 = call "Read Contour Display Rate (SubVI).vi"() -> ("Rate (Hz)"=w611:u32)  [unwired: 11 in]
      n455 = call "Read GALVO Calibration File (SubVI).vi"() -> ("GALVO Cal Data"=w591:T21)  [unwired: 11 in]
      n456 = local read "Command Q"() -> (w612:refnum<queue>)
      n457 = local write "Display Frame Rate (Hz)"(w611) -> ()
      n458 = call "Read DMD Calibration Files (SubVI).vi"() -> ("DMD2 Int"=w593:dbl[][], "DMD1 Int"=w594:dbl[][], "error out"=w596:errorcluster, "DMD1X"=w610:dbl[][], "DMD1Y"=w609:dbl[][], "DMD2X"=w608:dbl[][], "DMD2Y"=w595:dbl[][])  [unwired: 9 in]
      n459 = disable-structure shown="Disabled" {
        disable-tunnel: [w613 _] -> w597
        frame Disabled {
          n460 = Open/Create/Replace File(file path (use dialog)=path "C:/MWT/log.txt", operation (0:open)=T17."replace or create") -> (refnum out=w613:refnum<file>)  [unwired: 4 in, 2 out]
        }
        frame Enabled {
        }
      }
      n461 = call "Read DMD Calibration Parameter (SubVI).vi"() -> ("DMD Intensity Cal Param"=w592:T22)  [unwired: 11 in]
      n462 = Preview Queue Element(queue=w612) -> ()  [unwired: 2 in, 4 out]
      n463 = case shown="No Error" w596 {
        tunnel: w591 -> [_ _]
        frame No Error {
          "Files Loaded" <- TRUE ("TP")
        }
        frame Error {
        }
      }
      n464 = call "Initialize DMD 1 Control (SubVI).vi"() -> ("DMD IMG REF"=w603:refnum<vi>, "STOP REF"=w601:refnum<vi>, "DMD VI REF"=w600:refnum<vi>)  [unwired: 9 in]
      n465 = call "Initialize DMD 2 Control (SubVI).vi"() -> ("DMD IMG REF"=w602:refnum<vi>, "STOP REF"=w598:refnum<vi>, "DMD VI REF"=w599:refnum<vi>)  [unwired: 9 in]
      n466 = Initialize Array(0.0 ("element"), 768 ("dimension size"), 1024 ("dimension size")) -> (w604:dbl[][])
    }
    frame #1 {
      w624 = path "C:/Users/labadmin/Documents/projectContributors/Michael/multi-larva-cl-behavior-detection/LabViewSourceCode/heatCameraPythonCode/customFlir.py" ("module path")
      w681 = FALSE ("Save")
      # "Initialise Python session"
      # "INPUT current DMD input"
      # "From REF, insert Display Image to current code block"
      n467 = local read "REF"() -> (w665:T5)
      n468 = Unbundle By Name(w665) -> ("Queue REF.DMD Input"=w666:refnum<queue>)
      n469 = while {
        tunnel: w666 -> [w848]
        tunnel: w664 -> [w845]
        tunnel: w663 -> [w844]
        tunnel: w662 -> [w843]
        tunnel: w661 -> [w842]
        tunnel: w660 -> [w846]
        tunnel: w659 -> [w841]
        tunnel: w658 -> [w840]
        tunnel: w657 -> [w839]
        tunnel: w656 -> [w838]
        tunnel: [w837] -> w652
        tunnel: [w836] -> w649
        tunnel: w643 -> [w835]
        tunnel: [w834] -> w642
        tunnel: w641 -> [w823]
        stop <- w849 stop-if-true
        # "DMD Control Loop"
        n470 = Dequeue Element(queue=w848, timeout in ms (-1)=100) -> (element=w847:i32[], timed out?=w832:bool)  [unwired: 1 in, 2 out]
        n471 = case shown="False" w832 {
          tunnel: w847 -> [w851 _]
          tunnel: w846 -> [w869 _]
          tunnel: w845 -> [w867 _]
          tunnel: w844 -> [w866 _]
          tunnel: w843 -> [w865 _]
          tunnel: w842 -> [w864 _]
          tunnel: w841 -> [w863 _]
          tunnel: w840 -> [w862 _]
          tunnel: w839 -> [w857 _]
          tunnel: w838 -> [w856 _]
          tunnel: [w855 _] -> w837
          tunnel: [w854 _] -> w836
          tunnel: w835 -> [w853 w880]
          tunnel: [w852 w880] -> w834
          tunnel: w823 -> [w850 _]
          frame False {
            # "Get current DM stimulus parameters"
            # "Set DMD 2 REF to DMD 2 image"
            # "Set DMD 1 REF to DMD 1 image"
            n472 = local read "Pixel Resolution (um/Pixel)"() -> (w870:dbl)
            n473 = call "Rearrange DLL Output (SubVI).vi"("outData"=w851) -> ("Stimulus Parameters"=w868:dbl[][])  [unwired: 10 in]
            n474 = call "Construct DMD 1 Image (SubVI).vi"("DMD1X Array"=w867, "DMD1Y Array"=w866, "Stimulus Parameters"=w868, "DMD Intensity Cal Param"=w850, "Intensity Coefficients"=w863, "Pixel Resolution (um/Pixel)"=w870, "Initialized DMD Image Array"=w869) -> ("Image Array"=w859:u8[][])  [unwired: 12 in]
            n475 = call "Construct DMD 2 Image (SubVI).vi"("DMD2X Array"=w865, "DMD2Y Array"=w864, "Stimulus Parameters"=w868, "DMD Intensity Cal Param"=w850, "Intensity Coefficients"=w862, "Pixel Resolution (um/Pixel)"=w870, "Initialized DMD Image Array"=w869) -> ("Image Array"=w858:u8[][])  [unwired: 12 in]
            n476 = disable-structure shown="Disabled" {
              disable-tunnel: w853 -> [w876 _]
              disable-tunnel: [w874 _] -> w852
              frame Disabled {
                n477 = Get Date/Time In Seconds() -> (seconds since 1Jan1904=w875:timestamp)
                n478 = To Double Precision Float(number=w875) -> (double precision float=w871:dbl)
                n479 = feedback #3(w871) -> (w872:dbl)
                n480 = feedback-in #3(w871) -> ()
                n481 = Subtract(x=w871, y=w872) -> (x-y=w873:dbl)
                n482 = Number To Fractional String(number=w873) -> (F-format string=w877:string)  [unwired: 3 in]
                n483 = Concatenate Strings(w877, "\r\n") -> (w878:string)
                n484 = Write to Text File(file (use dialog)=w876, text=w878) -> (refnum out=w874:refnum<file>)  [unwired: 2 in, 2 out]
              }
              frame Enabled {
              }
            }
            n485 = To Variant(anything=w859) -> (Variant=w861:variant)
            n486 = To Variant(anything=w858) -> (Variant=w860:variant)
            n487 = property class="Ctl"(reference=w857, "Value"=w861) -> (error out=w855:errorcluster)  [unwired: 1 in, 1 out]
            n488 = property class="Ctl"(reference=w856, "Value"=w860) -> (error out=w854:errorcluster)  [unwired: 1 in, 1 out]
          }
          frame True {
          }
        }
        n489 = local read "Frame Rate"() -> (w825:u32)
        n490 = Greater Than 0?(x=w825) -> (x > 0?=w826:bool)
        n491 = Select(t=w825, s=w826, f=u32 1) -> (s? t:f=w827:u32)
        n492 = To Double Precision Float(number=w827) -> (double precision float=w831:dbl)
        n493 = Divide(x=1000.0, y=w831) -> (x/y=w829:dbl)
        n494 = To Unsigned Long Integer(number=w829) -> (unsigned 32bit integer=w828:u32)
        n495 = Wait Until Next ms Multiple(millisecond multiple=w828) -> ()  [unwired: 1 out]
        n496 = property on="Stopped?" class="Bool (strict)"() -> ("Value"=w849:bool)  [unwired: 2 in, 2 out]
      }
      n497 = disable-structure shown="Disabled" {
        disable-tunnel: w642 -> [w822 _]
        frame Disabled {
          n498 = Close File(refnum=w822) -> ()  [unwired: 1 in, 2 out]
        }
        frame Enabled {
        }
      }
      n499 = To Variant(anything=TRUE ("Wait Until Done")) -> (Variant=w654:variant)
      n500 = To Variant(anything=TRUE ("Wait Until Done")) -> (Variant=w647:variant)
      n501 = property class="Ctl"(reference=w651, error in=w652, "Value"=w654) -> (error out=w653:errorcluster)  [unwired: 1 out]
      n502 = property class="Ctl"(reference=w644, error in=w649, "Value"=w647) -> (error out=w648:errorcluster)  [unwired: 1 out]
      n503 = invoke class="VI" method="FP.Close"(reference=w650, error in=w653) -> ()  [unwired: 1 in, 3 out]
      n504 = invoke class="VI" method="FP.Close"(reference=w645, error in=w648) -> ()  [unwired: 1 in, 3 out]
      n505 = local read "REF"() -> (w668:T5)
      n506 = Unbundle By Name(w668) -> ("Queue REF.Display Image"=w669:refnum<queue>)
      n507 = call "Create AVI FName (SubVI).vi"("Save"=w681) -> ("Image REF"=w678:T8, "AVI Refnum"=w679:T15)  [unwired: 9 in]
      n508 = while {
        tunnel: [w1013] -> w667
        tunnel: w669 -> [w1012]
        tunnel: w679 -> [w1009]
        tunnel: [w1008] -> w671
        tunnel: w678 -> [w1007]
        tunnel: w681 -> [w1006]
        tunnel: w681 -> [w1005]
        stop <- w1010 stop-if-true
        # "Take an image and pass it on every 100 ms?"
        # "Case structure: is testing on?"
        # "Display Image"
        n509 = property on="Stopped?" class="Bool (strict)"() -> ("Value"=w1010:bool)  [unwired: 2 in, 2 out]
        n510 = Dequeue Element(queue=w1012, timeout in ms (-1)=100) -> (queue out=w1014:refnum<queue>, element=w1011:T16, timed out?=w1015:bool)  [unwired: 1 in, 1 out]
        n511 = case shown="False" w1015 {
          tunnel: w1014 -> [w1024 w1097]
          tunnel: [w1024 w1097] -> w1013
          tunnel: w1011 -> [w1023 _]
          tunnel: w1009 -> [w1022 w1096]
          tunnel: [w1021 w1096] -> w1008
          tunnel: w1007 -> [w1020 _]
          tunnel: w1006 -> [w1018 _]
          tunnel: w1005 -> [w1017 _]
          frame False {
            # "MAIN PROGRAM CODE"
            # "Testing code to save progam GUI screeshots to .avi"
            n512 = flat-sequence {
              tunnel: w1023 -> [w1031]
              tunnel: [w1091] -> w1019
              tunnel: w1017 -> [w1090]
              frame #0 {
                # "Only if > 0"
                # "Set (slow) frame rate for displaying larva outlines (default = 5 Hz)"
                # "DISPLAY DETECTED LARVA OUTLINES / SPINES"
                # "Display image"
                # "SHOW LIVE / BG / BG-SUBTRACTED IMAGE\nCase structure which determines what image will be displayed, based on input from Display Type"
                # "GUI button to select display type"
                n513 = Greater Than 0?(x="Display Frame Rate (Hz)") -> (x > 0?=w1034:bool)
                n514 = case shown="True" w1034 {
                  tunnel: w1031 -> [_ w1066]
                  tunnel: "Display Frame Rate (Hz)" -> [_ w1056]
                  frame False {
                  }
                  frame True {
                    # "Take display data and return contour, spine, head, tail, and ID data"
                    # "For loop to display larva outlines (1-8)"
                    # "Calculate ms to wait (from Hz)"
                    # "Convert to double precision"
                    n515 = call "Display Contour SPINE Head Tail (SubVI).vi"("Display Data"=w1066) -> ("Contour Array"=w1065:cluster{"Array":i32[], "Array":i32[]}[], "SPINE Array"=w1064:cluster{"Array":i32[], "Array":i32[]}[], "Head Array"=w1063:cluster{"Array":i32[], "Array":i32[]}[], "Tail Array"=w1062:cluster{"Array":i32[], "Array":i32[]}[], "Larvae ID"=w1061:u32[])  [unwired: 10 in]
                    n516 = for {
                      tunnel: w1065 -> [w1073] mode=indexing
                      tunnel: w1064 -> [w1072] mode=indexing
                      tunnel: w1063 -> [w1071] mode=indexing
                      tunnel: w1062 -> [w1070] mode=indexing
                      tunnel: w1061 -> [w1067] mode=indexing
                      i -> [w1068]
                      # "i = iteration count"
                      # "Combine outlines/spines/etc data into single array"
                      n517 = Build Array(w1073, w1072, w1071, w1070) -> (w1069:cluster{"Array":i32[], "Array":i32[]}[])
                      n518 = case shown="2" w1068 {
                        tunnel: w1069 -> [w1075 w1077 w1079 w1081 w1083 w1085 w1087 w1089 _]
                        tunnel: w1067 -> [w1074 w1076 w1078 w1080 w1082 w1084 w1086 w1088 _]
                        frame 0 {
                          # "Show outlines"
                          # "Show larva ID"
                          "Larvae 1" <- w1075
                          "Larvae 1" <- w1074
                        }
                        frame 1 {
                          "Larvae 2" <- w1077
                          "Larvae 2" <- w1076
                        }
                        frame 2 {
                          "Larvae 3" <- w1079
                          "Larvae 3" <- w1078
                        }
                        frame 3 {
                          "Larvae 4" <- w1081
                          "Larvae 4" <- w1080
                        }
                        frame 4 {
                          "Larvae 5" <- w1083
                          "Larvae 5" <- w1082
                        }
                        frame 5 {
                          "Larvae 6" <- w1085
                          "Larvae 6" <- w1084
                        }
                        frame 6 {
                          "Larvae 7" <- w1087
                          "Larvae 7" <- w1086
                        }
                        frame 7 {
                          "Larvae 8" <- w1089
                          "Larvae 8" <- w1088
                        }
                        frame 8, Default {
                        }
                      }
                    }
                    n519 = To Double Precision Float(number=w1056) -> (double precision float=w1057:dbl)
                    n520 = Divide(x=1000.0, y=w1057) -> (x/y=w1058:dbl)
                    n521 = To Unsigned Long Integer(number=w1058) -> (unsigned 32bit integer=w1060:u32)
                    n522 = Wait (ms)(milliseconds to wait=w1060) -> ()  [unwired: 1 out]
                  }
                }
                n523 = case shown="\"Background-Live\"" "Display Type" {
                  tunnel: w1031 -> [w1036 _ w1054]
                  tunnel: [w1035 w1038 w1049] -> w1030
                  frame "Live", Default {
                    # "Get live image data and return final image object"
                    n524 = local read "Image Size"() -> (w1037:T3)
                    n525 = call "Display Preview (SubVI).vi"("Display Data"=w1036, "Image Size"=w1037) -> ("Image Out"=w1035:T8)  [unwired: 17 in]
                  }
                  frame "Background" {
                    # "Produce BG image object"
                    # "Insert BG image data"
                    # "Create an image called BG1"
                    n526 = local read "BG Image"() -> (w1040:u8[][])
                    n527 = call "IMAQ Create"("Image Name"="BG1") -> ("New Image"=w1039:T8)  [unwired: 4 in, 1 out]
                    n528 = call "IMAQ ArrayToImage"("Image Pixels (U8)"=w1040, "Image"=w1039) -> ("Image Out"=w1038:T8)  [unwired: 8 in, 1 out]
                  }
                  frame "Background-Live" {
                    # "\"READ\" local variable"
                    n529 = Unbundle By Name(w1054) -> ("Image Data"=w1053:u64[])
                    n530 = local read "Image Size"() -> (w1048:T3)
                    n531 = local read "BG Image"() -> (w1055:u8[][])
                    n532 = call "Convert Array to Image (SubVI).vi"("Image Size"=w1048, "Image Array In"=w1053) -> ("Image Array Out"=w1052:u8[][])  [unwired: 9 in]
                    n533 = To Word Integer(number=w1055) -> (16bit integer=w1043:i16[][])
                    n534 = To Word Integer(number=w1052) -> (16bit integer=w1044:i16[][])
                    n535 = Subtract(x=w1043, y=w1044) -> (x-y=w1051:i16[][])
                    n536 = In Range and Coerce(upper limit=i16 255, x=w1051, lower limit=i16 0) -> (coerced(x)=w1047:i16[][])  [unwired: 1 out]
                    n537 = To Unsigned Byte Integer(number=w1047) -> (unsigned 8bit integer=w1042:u8[][])
                    n538 = call "IMAQ Create"("Image Name"="BG-SUB") -> ("New Image"=w1049:T8)  [unwired: 4 in, 1 out]
                    n539 = call "IMAQ ArrayToImage"("Image Pixels (U8)"=w1042, "Image"=w1049) -> ()  [unwired: 8 in, 2 out]
                  }
                }
                "Display" <- w1030
              }
              frame #1 {
                # "Here, an invoke node is used to run the current VI. The method run is \"FP.Get Image\", with parmeters: Visible Area Only and Image Depth. The output of the function is Image Data (which is then sent for saving to .avi if testing is turned on"
                n540 = case shown="True" w1090 {
                  tunnel: [_ w1095] -> w1091
                  frame False {
                  }
                  frame True {
                    n541 = control-ref of="This VI"() -> (w1094:refnum<vi>)
                    n542 = invoke class="VI" method="FP.Get Image"(reference=w1094, "visible area only"=TRUE ("Visible Area Only"), "image depth"=24 ("Image Depth")) -> ("image data"=w1095:T23)  [unwired: 3 in, 5 out]
                  }
                }
              }
            }
            n543 = case shown="True" w1018 {
              tunnel: w1022 -> [_ w1029]
              tunnel: [_ w1028] -> w1021
              tunnel: w1020 -> [_ w1027]
              tunnel: w1019 -> [_ w1026]
              frame False {
              }
              frame True {
                n544 = call "Convert LabVIEW Image Data To IMAQ.vi"("Image Data"=w1026, "Image In"=w1027) -> ("Image Out"=w1025:T8)  [unwired: 8 in, 1 out]
                n545 = call "IMAQ AVI2 Write Frame"("Image"=w1025, "AVI Refnum"=w1029) -> ("AVI Refnum (duplicate)"=w1028:T15)  [unwired: 7 in, 2 out]
              }
            }
          }
          frame True {
          }
        }
      }
      n546 = case shown="True" w681 {
        tunnel: w671 -> [_ w881]
        frame False {
        }
        frame True {
          n547 = call "IMAQ AVI2 Close"("AVI Refnum"=w881) -> ()  [unwired: 10 in, 1 out]
        }
      }
      n548 = Release Queue(queue=w667) -> (error out=w680:errorcluster)  [unwired: 2 in, 2 out]
      n549 = call <vilib>:"Clear Errors.vi"("error in (no error)"=w680) -> ()  [unwired: 5 in, 2 out]
      n550 = local read "REF"() -> (w676:T5)
      n551 = Unbundle By Name(w676) -> ("FPGA REF (MWT)"=w677:T7, "Queue REF.Tag Image"=w675:refnum<queue>)
      n552 = while {
        tunnel: [w886] -> w674
        tunnel: w675 -> [w885]
        tunnel: w677 -> [w882]
        stop <- w883 stop-if-true
        # "Larvae Identification"
        n553 = property on="Stopped?" class="Bool (strict)"() -> ("Value"=w883:bool)  [unwired: 2 in, 2 out]
        n554 = Dequeue Element(queue=w885, timeout in ms (-1)=100) -> (queue out=w887:refnum<queue>, element=w884:T16, timed out?=w888:bool)  [unwired: 1 in, 1 out]
        n555 = case shown="False" w888 {
          tunnel: w887 -> [w906 w907]
          tunnel: [w906 w907] -> w886
          tunnel: w884 -> [w904 _]
          tunnel: w882 -> [w894 _]
          frame False {
            # "Send identified bounding boxes to FPGA"
            n556 = local read "Pixel Intensity Range"() -> (w902:cluster{"Low":u8, "High":u8})
            n557 = local read "Subtract BG"() -> (w897:bool)
            n558 = local read "Image Size"() -> (w903:T3)
            n559 = local read "BG SUB TH"() -> (w896:i16)
            n560 = local read "BG Image"() -> (w898:u8[][])
            n561 = local read "flipFlag"() -> (w890:refnum<queue>)
            n562 = local read "vReset"() -> (w891:refnum<queue>)
            n563 = call "Re-tag Larvae v2 (SubVI).vi"("Image Size"=w903, "BG SUB TH"=w896, "Subtract BG"=w897, "BG Image"=w898, "vReset"=w891, "Data In"=w904, "Range"=w902, "flipFlag"=w890, "Box Side"="Box Side (Pixels)", "Box W + L"="Box W + L (Pixels)", "Area"="Area (Pixels)") -> ("# of Objects"=→"# Objects":i32, "BBOX Array"=w893:u64[], "HT LOC"=w892:u64[])  [unwired: 6 in]
            n564 = Wait (ms)(milliseconds to wait=u32 50) -> ()  [unwired: 1 out]
            n565 = call "Send Block and HT Position (SubVI).vi"("HT LOC"=w892, "BBOX Array"=w893, "FPGA REF"=w894) -> ()  [unwired: 9 in]
          }
          frame True {
          }
        }
      }
      n566 = Release Queue(queue=w674) -> (error out=w682:errorcluster)  [unwired: 2 in, 2 out]
      n567 = local read "REF"() -> (w632:T5)
      n568 = call <vilib>:"Clear Errors.vi"("error in (no error)"=w682) -> ()  [unwired: 5 in, 2 out]
      n569 = Unbundle By Name(w632) -> ("Queue REF.Save Image"=w631:refnum<queue>)
      n570 = local read "REF"() -> (w673:T5)
      n571 = case shown="True" FALSE {
        frame False {
        }
        frame True {
          # "Setup binary file"
          # "Setup AVI with given codec"
          n572 = local read "REF"() -> (w781:T5)
          n573 = local read "Exp. Time (S)"() -> (w775:dbl)
          n574 = Unbundle By Name(w781) -> ("Queue REF.Display Image"=w780:refnum<queue>)
          n575 = property on="Stopped?" class="Bool (strict)"() -> ("Value"=w770:bool)  [unwired: 2 in, 2 out]
          n576 = Greater?(x=w775, y=0.0) -> (0:w771:bool)
          n577 = call "IMAQ AVI2 Create"("Codec"="Motion JPEG (NI Vision)" ("CODEC"), "Frames Per Second"=u32 25, "AVI Path"=path "C:/Users/labadmin/Documents/projectContributors/Michael/sampleData.avi") -> ("AVI Refnum"=w776:T15)  [unwired: 7 in, 1 out]
          n578 = Not Equal?(x=w770, y=TRUE) -> (x != y?=w772:bool)
          n579 = And(x=w772, y=w771) -> (x .and. y?=w769:bool)
          n580 = call "IMAQ Create"("Image Name"="curImage") -> ("New Image"=w783:T8)  [unwired: 4 in, 1 out]
          n581 = while {
            tunnel: w783 -> [w789]
            tunnel: w780 -> [w785]
            tunnel: w776 -> [w788]
            tunnel: w769 -> [w786]
            tunnel: [w785] -> w767
            tunnel: path "C:/Users/labadmin/Documents/projectContributors/Michael/sampleData.bin" ("file (use dialog)") -> [w784]
            stop <- w787 stop-if-true
            # "Save current camera image to AVI"
            n582 = property on="Stopped?" class="Bool (strict)"() -> ("Value"=w787:bool)  [unwired: 2 in, 2 out]
            n583 = case shown="True" w786 {
              tunnel: w789 -> [_ w795]
              tunnel: w785 -> [_ w794]
              tunnel: w788 -> [_ w792]
              tunnel: w784 -> [_ w791]
              frame False {
              }
              frame True {
                n584 = Dequeue Element(queue=w794, timeout in ms (-1)=100) -> (element=w800:T16)  [unwired: 1 in, 3 out]
                n585 = Unbundle By Name(w800) -> ("Image Data"=w799:u64[])
                n586 = local read "Image Size"() -> (w798:T3)
                n587 = call "Convert Array to Image (SubVI).vi"("Image Size"=w798, "Image Array In"=w799) -> ("Image Array Out"=w790:u8[][])  [unwired: 9 in]
                n588 = Write to Binary File(file (use dialog)=w791, data=w790) -> ()  [unwired: 4 in, 3 out]
                n589 = local read "Stopped?"() -> (w793:bool)
                n590 = call "IMAQ ArrayToImage"("Image Pixels (U8)"=w790, "Image"=w795) -> ("Image Out"=w797:T8)  [unwired: 8 in, 1 out]
                n591 = case shown="True" w793 {
                  tunnel: w792 -> [_ w801]
                  frame False {
                  }
                  frame True {
                    n592 = call "IMAQ AVI2 Close"("AVI Refnum"=w801) -> ()  [unwired: 10 in, 1 out]
                  }
                }
                n593 = call "IMAQ AVI2 Write Frame"("Image"=w797, "AVI Refnum"=w792) -> ()  [unwired: 7 in, 3 out]
              }
            }
          }
          n594 = Release Queue(queue=w767) -> (error out=w768:errorcluster)  [unwired: 2 in, 2 out]
          n595 = call <vilib>:"Clear Errors.vi"("error in (no error)"=w768) -> ()  [unwired: 5 in, 2 out]
        }
      }
      n596 = Unbundle By Name(w673) -> ("Queue REF.BG Image"=w672:refnum<queue>)
      n597 = while {
        tunnel: w631 -> [w718]
        tunnel: [w715] -> w629
        shift-right: [w716] -> w630
        shift-left: _ -> [w711]
        stop <- w717 stop-if-true
        # "Save live image as binary file"
        n598 = property on="Stopped?" class="Bool (strict)"() -> ("Value"=w717:bool)  [unwired: 2 in, 2 out]
        n599 = Dequeue Element(queue=w718, timeout in ms (-1)=100) -> (element=w713:T16, timed out?=w712:bool)  [unwired: 1 in, 2 out]
        n600 = case shown="False" w712 {
          tunnel: [w738 w765] -> w716
          tunnel: [w737 _] -> w715
          tunnel: w713 -> [w736 _]
          tunnel: w711 -> [_ w765]
          frame False {
            w719 = T20."little-endian" ("byte order (0:big-endian, network order)")
            # "Frame # and Time stamp"
            n601 = feedback #4(TRUE) -> (w734:bool)
            n602 = feedback-in #4(FALSE) -> ()
            n603 = feedback #5() -> (w732:refnum<file>)  [unwired: 1 in]
            n604 = case shown="True" w734 {
              tunnel: [w739 w754] -> w731
              tunnel: w732 -> [w739 _]
              frame False {
              }
              frame True {
                # "UNUSED"
                n605 = Get Date/Time In Seconds() -> (seconds since 1Jan1904=w758:timestamp)
                n606 = Format Date/Time String(time format string (%c)="%H%M%S", seconds (now)=w758) -> ()  [unwired: 1 in, 1 out]
                n607 = local read "FNP"() -> (w751:T1)
                n608 = Unbundle By Name(w751) -> ("DateTimeStamp"=w750:string)
                n609 = Build Path(base path="File Path", name or relative path=w750) -> (appended path=w760:path)
                n610 = call <vilib>:"Check if File or Folder Exists.vi"("path"=w760) -> ("file or folder exists?"=w757:bool, "dup path"=w749:path)  [unwired: 8 in, 1 out]
                n611 = Build Path(base path=w749, name or relative path=path "bg.BGimage") -> (appended path=w747:path)
                n612 = case shown="False" w757 {
                  tunnel: w749 -> [w763 w764]
                  tunnel: [w762 w764] -> w752
                  frame False {
                    n613 = Create Folder(path (use dialog)=w763) -> (created path=w762:path)  [unwired: 2 in, 2 out]
                  }
                  frame True {
                  }
                }
                n614 = Open/Create/Replace File(file path (use dialog)=w747, operation (0:open)=T17."open or create") -> (refnum out=w743:refnum<file>)  [unwired: 4 in, 2 out]
                n615 = local read "BG Image"() -> (w745:u8[][])
                n616 = Write to Binary File(file (use dialog)=w743, data=w745, 5:FALSE ("prepend array or string size? (T)"), 9:T20."little-endian" ("byte order (0:big-endian, network order)")) -> (refnum out=w740:refnum<file>, error out=w741:errorcluster)  [unwired: 2 in, 1 out]
                n617 = Build Path(base path=w752, name or relative path="video.bin") -> (appended path=w761:path)
                n618 = Close File(refnum=w740, error in=w741) -> ()  [unwired: 2 out]
                n619 = Open/Create/Replace File(file path (use dialog)=w761, operation (0:open)=T17."open or create") -> (refnum out=w754:refnum<file>)  [unwired: 4 in, 2 out]
              }
            }
            n620 = feedback-in #5(w731) -> ()
            n621 = Unbundle By Name(w736) -> ("Frame Number"=w725:u64, "Time Stamp (us)"=w722:u64)
            n622 = Unbundle By Name(w736) -> ("Image Data"=w730:u64[])
            n623 = local read "Image Size"() -> (w728:T3)
            n624 = Write to Binary File(file (use dialog)=w731, data=w725, 5:FALSE ("prepend array or string size? (T)"), 9:w719) -> (refnum out=w723:refnum<file>)  [unwired: 2 in, 2 out]
            n625 = Write to Binary File(file (use dialog)=w723, data=w722, 5:FALSE ("prepend array or string size? (T)"), 9:w719) -> (refnum out=w721:refnum<file>)  [unwired: 2 in, 2 out]
            n626 = Write to Binary File(file (use dialog)=w721, data=w728, 5:FALSE ("prepend array or string size? (T)"), 9:w719) -> (refnum out=w726:refnum<file>)  [unwired: 2 in, 2 out]
            n627 = Write to Binary File(file (use dialog)=w726, data=w730, 5:FALSE ("prepend array or string size? (T)"), 9:w719) -> (refnum out=w738:refnum<file>, error out=w737:errorcluster)  [unwired: 2 in, 1 out]
          }
          frame True {
          }
        }
      }
      n628 = while {
        shift-right: [w913] -> _
        shift-left: Capture_Background_Image."Download Image" -> [w914]
        shift-right: [w912] -> _
        shift-left: _ -> [w911]
        tunnel: w672 -> [w908]
        shift-right: [w910] -> _
        shift-left: _ -> [w909]
        tunnel: [w908] -> w684
        stop <- w915 stop-if-true
        # "Background Image Capture"
        n629 = case shown="\"Save Image\"" w914 {
          selector: w914 -> [_ w940 _ _]
          tunnel: [w921 w941 Capture_Background_Image."Download Image" Capture_Background_Image."Wait for UI"] -> w913
          tunnel: [0 w942 w986 _] -> w912
          tunnel: w911 -> [_ w943 w986 _]
          tunnel: w908 -> [_ w945 _ w996]
          tunnel: [w917 w938 w975 w987] -> w910
          tunnel: w909 -> [w916 w937 w975 _]
          frame "Wait for UI", Default {
            n630 = case shown="True" "Capture BG" {
              tunnel: [w925 w934] -> w917
              tunnel: w916 -> [w925 _]
              frame False {
                n631 = property on="Capture BG" class="Bool (strict)"("DisabledEnum"=T9."Enabled" ("Disabled")) -> ()  [unwired: 2 in, 2 out]
              }
              frame True {
                n632 = local read "Image Size"() -> (w933:T3)
                n633 = property on="Capture BG" class="Bool (strict)"("DisabledEnum"=T9."Disabled" ("Disabled")) -> ()  [unwired: 2 in, 2 out]
                n634 = To Long Integer(number=w933) -> (32bit integer=w932:cluster{"Height":i32, "Width":i32})
                n635 = Unbundle By Name(w932) -> ("Height"=w931:i32, "Width"=w930:i32)
                n636 = Select(t=u8 0, s="BG Type", f=u8 255 ("element")) -> (s? t:f=w928:u8)
                n637 = Initialize Array(w928, w931, w930) -> (w934:u8[][])
              }
            }
            n638 = Select(t=Capture_Background_Image."Acquire Image", s="Capture BG", f=Capture_Background_Image."Wait for UI") -> (s? t:f=w921:T19)
            n639 = Wait (ms)(milliseconds to wait=u32 100) -> ()  [unwired: 1 out]
          }
          frame "Acquire Image" {
            n640 = Dequeue Element(queue=w945, timeout in ms (-1)=100) -> (element=w939:u64[], timed out?=w944:bool)  [unwired: 1 in, 2 out]
            n641 = case shown="False" w944 {
              tunnel: w943 -> [w965 w974]
              tunnel: [w961 w974] -> w942
              tunnel: [w962 w973] -> w941
              tunnel: w940 -> [_ w973]
              tunnel: w939 -> [w958 _]
              tunnel: [w947 w972] -> w938
              tunnel: w937 -> [w954 w972]
              frame False {
                n642 = Increment(x=w965) -> (x+1=w961:i32)
                n643 = local read "Image Size"() -> (w952:T3)
                n644 = To Long Integer(number=w952) -> (32bit integer=w951:cluster{"Height":i32, "Width":i32})
                n645 = Unbundle By Name(w951) -> ("Height"=w949:i32, "Width"=w950:i32)
                n646 = Flatten To String(anything=w958, prepend array or string size? (T)=FALSE, byte order (0:big-endian, network order)=T20."little-endian") -> (data string=w956:string)  [unwired: 1 in, 2 out]
                n647 = String To Byte Array(string=w956) -> (unsigned byte array=w955:u8[])
                n648 = local read "BG Type"() -> (w946:bool)
                n649 = Reshape Array(w955, w949, w950) -> (w953:u8[][])
                n650 = case shown="False" w946 {
                  tunnel: w954 -> [w968 w971]
                  tunnel: w953 -> [w967 w970]
                  tunnel: [w966 w969] -> w947
                  frame True {
                    n651 = Max & Min(x=w967, y=w968) -> (max(x,y)=w966:u8[][])  [unwired: 1 out]
                  }
                  frame False {
                    n652 = Max & Min(x=w970, y=w971) -> (min(x,y)=w969:u8[][])  [unwired: 1 out]
                  }
                }
                n653 = Greater?(x=w961, y=250) -> (0:w960:bool)
                n654 = Select(t=Capture_Background_Image."Save Image", s=w960, f=Capture_Background_Image."Acquire Image") -> (s? t:f=w962:T19)
              }
              frame True {
              }
            }
          }
          frame "Save Image" {
            n655 = local write "Capture BG"(FALSE ("Capture BG")) -> ()
            n656 = call <vilib>:"Application Directory.vi"() -> ("Application Directory"=w984:path)
            n657 = Build Path(base path=w984, name or relative path="BGImage.bin") -> (appended path=w982:path)
            n658 = Open/Create/Replace File(file path (use dialog)=w982, operation (0:open)=T17."replace or create") -> (refnum out=w980:refnum<file>)  [unwired: 4 in, 2 out]
            n659 = Write to Binary File(file (use dialog)=w980, data=w975, 5:FALSE ("prepend array or string size? (T)")) -> (refnum out=w977:refnum<file>, error out=w978:errorcluster)  [unwired: 3 in, 1 out]
            n660 = Close File(refnum=w977, error in=w978) -> ()  [unwired: 2 out]
          }
          frame "Download Image" {
            n661 = Flush Queue(queue=w996) -> ()  [unwired: 1 in, 3 out]
            n662 = call <vilib>:"Application Directory.vi"() -> ("Application Directory"=w1003:path)
            n663 = Build Path(base path=w1003, name or relative path="BGImage.bin") -> (appended path=w1001:path)
            n664 = local read "Image Size"() -> (w992:T3)
            n665 = Open/Create/Replace File(file path (use dialog)=w1001) -> (refnum out=w1000:refnum<file>)  [unwired: 5 in, 2 out]
            n666 = To Long Integer(number=w992) -> (32bit integer=w991:cluster{"Height":i32, "Width":i32})
            n667 = Get File Size(file=w1000) -> (refnum out=w999:refnum<file>, size (in bytes)=w998:i64)  [unwired: 1 in, 1 out]
            n668 = To Long Integer(number=w998) -> (32bit integer=w993:i32)
            n669 = Unbundle By Name(w991) -> ("Height"=w989:i32, "Width"=w990:i32)
            n670 = Read from Binary File(5:u8 0, 10:w993, 11:w999) -> (0:w995:errorcluster, 2:w988:u8[], 3:w994:refnum<file>)  [unwired: 3 in, 1 out]
            n671 = Reshape Array(w988, w989, w990) -> (w987:u8[][])
            "BG Image" <- w987
            n672 = Close File(refnum=w994, error in=w995) -> ()  [unwired: 2 out]
          }
        }
        n673 = property on="Stopped?" class="Bool (strict)"() -> ("Value"=w915:bool)  [unwired: 2 in, 2 out]
      }
      n674 = Release Queue(queue=w684) -> (error out=w683:errorcluster)  [unwired: 2 in, 2 out]
      n675 = call <vilib>:"Clear Errors.vi"("error in (no error)"=w683) -> ()  [unwired: 5 in, 2 out]
      n676 = Close File(refnum=w630, error in=w629) -> ()  [unwired: 2 out]
      n677 = local read "REF"() -> (w636:T5)
      n678 = Unbundle By Name(w636) -> ("Queue REF.GALVO Input"=w638:refnum<queue>)
      n679 = Open Python Session(python version="3.9" ("Python version")) -> (session out=w623:refnum<k35>)  [unwired: 2 in, 1 out]
      n680 = call "Initialize IR GALVO DAQ (SubVI).vi"() -> ("Refnum out"=w640:refnum<k21>)  [unwired: 11 in]
      n681 = while {
        shift-right: [w808] -> w639
        shift-left: w640 -> [w809]
        tunnel: w638 -> [w807]
        tunnel: [w803] -> w637
        tunnel: w634 -> [w802]
        stop <- w810 stop-if-true
        # "IR Stimulus Control"
        n682 = property on="Stopped?" class="Bool (strict)"() -> ("Value"=w810:bool)  [unwired: 2 in, 2 out]
        n683 = Dequeue Element(queue=w807, timeout in ms (-1)=50) -> (queue out=w803:refnum<queue>, element=w806:i32[], timed out?=w804:bool)  [unwired: 1 in, 1 out]
        n684 = case shown="False" w804 {
          tunnel: w809 -> [w817 w821]
          tunnel: [w819 w821] -> w808
          tunnel: w806 -> [w811 _]
          tunnel: w802 -> [w814 _]
          frame False {
            n685 = call "IR Stimulus DLL (SubVI).vi"("GALVO Calibration Data"=w814, "Cycle Time (ms)"="Cycle Time (ms)", "LASER Intensity (%)"="LASER Intensity (%)", "irData"=w811) -> ("Max. LASER Power (W)"=→"Max. LASER Power (W)":dbl, "daqData"=w816:dbl[][])  [unwired: 6 in]
            n686 = call-poly <vilib>:"DAQmx Write.vi"("task/channels in"=w817, "auto start"=TRUE, "data"=w816, "timeout"=1.0) -> ("task out"=w819:refnum<k21>)  [unwired: 9 in, 2 out]
          }
          frame True {
          }
        }
      }
      n687 = node(w623, w624, "setTemperatureRange" ("function name"), "Temperature Range (Low)", "Temperature Range (High)") -> ()  [unwired: 5 in, 4 out]
      n688 = while {
        tunnel: w624 -> [w702]
        tunnel: w623 -> [w701]
        tunnel: "getImage" ("function name") -> [w700]
        tunnel: "Array Type" -> [w699]
        tunnel: 640 ("dimension size") -> [w696]
        tunnel: 480 ("dimension size") -> [w695]
        stop <- FALSE stop-if-true
        n689 = Wait (ms)(milliseconds to wait=u32 100) -> ()  [unwired: 1 out]
        n690 = node(w701, w702, w700, w699) -> (w694:dbl[])  [unwired: 1 in, 4 out]
        n691 = Reshape Array(w694, w695, w696) -> (w688:dbl[][])
        n692 = for {
          tunnel: w688 -> [w710] mode=indexing
          tunnel: [w703] -> w691 mode=indexing
          n693 = local read "Temperature Range (High)"() -> (w707:dbl)
          n694 = local read "Temperature Range (Low)"() -> (w705:dbl)
          n695 = Divide(x=w710, y=255.0) -> (x/y=w708:dbl[])
          n696 = Subtract(x=w707, y=w705) -> (x-y=w706:dbl)
          n697 = Multiply(x=w706, y=w708) -> (x*y=w704:dbl[])
          n698 = Add(x=w705, y=w704) -> (x+y=w703:dbl[])
        }
        n699 = Reshape Array(w691, 480 ("dimension size"), 640 ("dimension size")) -> (w692:dbl[][])
        n700 = Transpose 2D Array(2D array=w692) -> (transposed array=→"Intensity Graph":dbl[][])
      }
      n701 = while {
        stop <- FALSE stop-if-true
        # "Login to heat camera stream every 20 seconds..."
        n702 = call <vilib>:"GET.vi"("url"="http://169.254.253.219/liveonly/admin:admin") -> ()  [unwired: 11 in, 4 out]
        n703 = Wait (ms)(milliseconds to wait=u32 20000) -> ()  [unwired: 1 out]
      }
      n704 = call <vilib>:"DAQmx Stop Task.vi"("task/channels in"=w639) -> ()  [unwired: 13 in, 2 out]
      n705 = Release Queue(queue=w637) -> (error out=w635:errorcluster)  [unwired: 2 in, 2 out]
      n706 = call <vilib>:"Clear Errors.vi"("error in (no error)"=w635) -> ()  [unwired: 5 in, 2 out]
      n707 = call "GetPalleteColors(SubVI).vi"("Map Selector"=T18."rainbow") -> ("Map output"=w617:u32[])  [unwired: 10 in]
      n708 = property on="Intensity Graph" class="IntGraph (strict)"("Color Table"=w617) -> ()  [unwired: 2 in, 2 out]
    }
  }
  n709 = local read "REF"() -> (w3:T5)
  n710 = disable-structure shown="Disabled" {
    disable-tunnel: w3 -> [w1098 _]
    frame Disabled {
      n711 = Unbundle By Name(w1098) -> ()  [unwired: 1 out]
      n712 = while {
        stop <- w1099 stop-if-true
        # "Enque DLL"
        n713 = property on="Stopped?" class="Bool (strict)"() -> ("Value"=w1099:bool)  [unwired: 2 in, 2 out]
      }
    }
    frame Enabled {
    }
  }
